vi "WSVCAP SHL FPGA TL Top Level.vi"() -> ()   [LabVIEW 2012]
uses:
  Type Defs/WSVCAP SHL State.ctl
  Type Defs/WSVCAP SHL Transaction Enum.ctl
  Type Defs/WSVCAP SHL Communication Loop State.ctl
  Type Defs/WSVCAP SHL FIFO Operation Enum.ctl
  Type Defs/WSVCAP SHL Operation Step Enum.ctl
  Type Defs/WSVCAP SHL Procedure Step Enum.ctl
  Type Defs/WSVCAP SHL Transaction Step Enum.ctl
  <vilib>/Platform/TimedLoop/XDataNode/timing_clust.ctl
  <vilib>/Platform/TimedLoop/XDataNode/nitl_modes.ctl
  <vilib>/Platform/TimedLoop/XDataNode/wakeup.ctl
  WSVCAP Shell FPGA Low Level/WSVCAP SHL FPGA LL RFFE Debug Global.vi
  WSVCAP Shell FPGA Low Level/WSVCAP SHL FPGA LL SPI Debug Global.vi
  WSVCAP Shell FPGA Low Level/WSVCAP SHL FPGA LL I2C Debug Global.vi
  <vilib>/Platform/TimedLoop/XDataNode/XDataNode.xnode
  <vilib>/Platform/TimedLoop/XDataNode/XDNodeRunTimeDep.lvlib
panel:
  in  "Stop Cycle":bool
  out "Cycle Count":u64
  in  "Socket Mask":u64=1 format="%012x"
  in  "Display CH (1-48)":i32=1 min=1 max=48 step=1
  out "Status":i32
  out "Read Data":u64
  in  "Transaction":T1
  in  "Bytes to Write":u8=8
  in  "Sub Address":u8=1 format="%02x"
  in  "Ack Read Status":bool
  out "Read Status Flag":bool
  in  "Exit":bool
  out "Waveform Chart":cluster{i16, i16, i16, i16}(graph)
  in  "Wait Ticks":u32=20
  in  "Slave Address":u8=1 format="%02x"
  in  "Bytes to Read":u8=8
  in  "Start":bool
  in  "Cmd":T2
  in  "Ack Read":bool
  out "Read Flag":bool
  in  "Write Flag":bool
  in  "Write Data":u64
  # "Control"
  # "I2C Configuration Parameters"
  # "Host Data Transfer"
  # "Command Type"
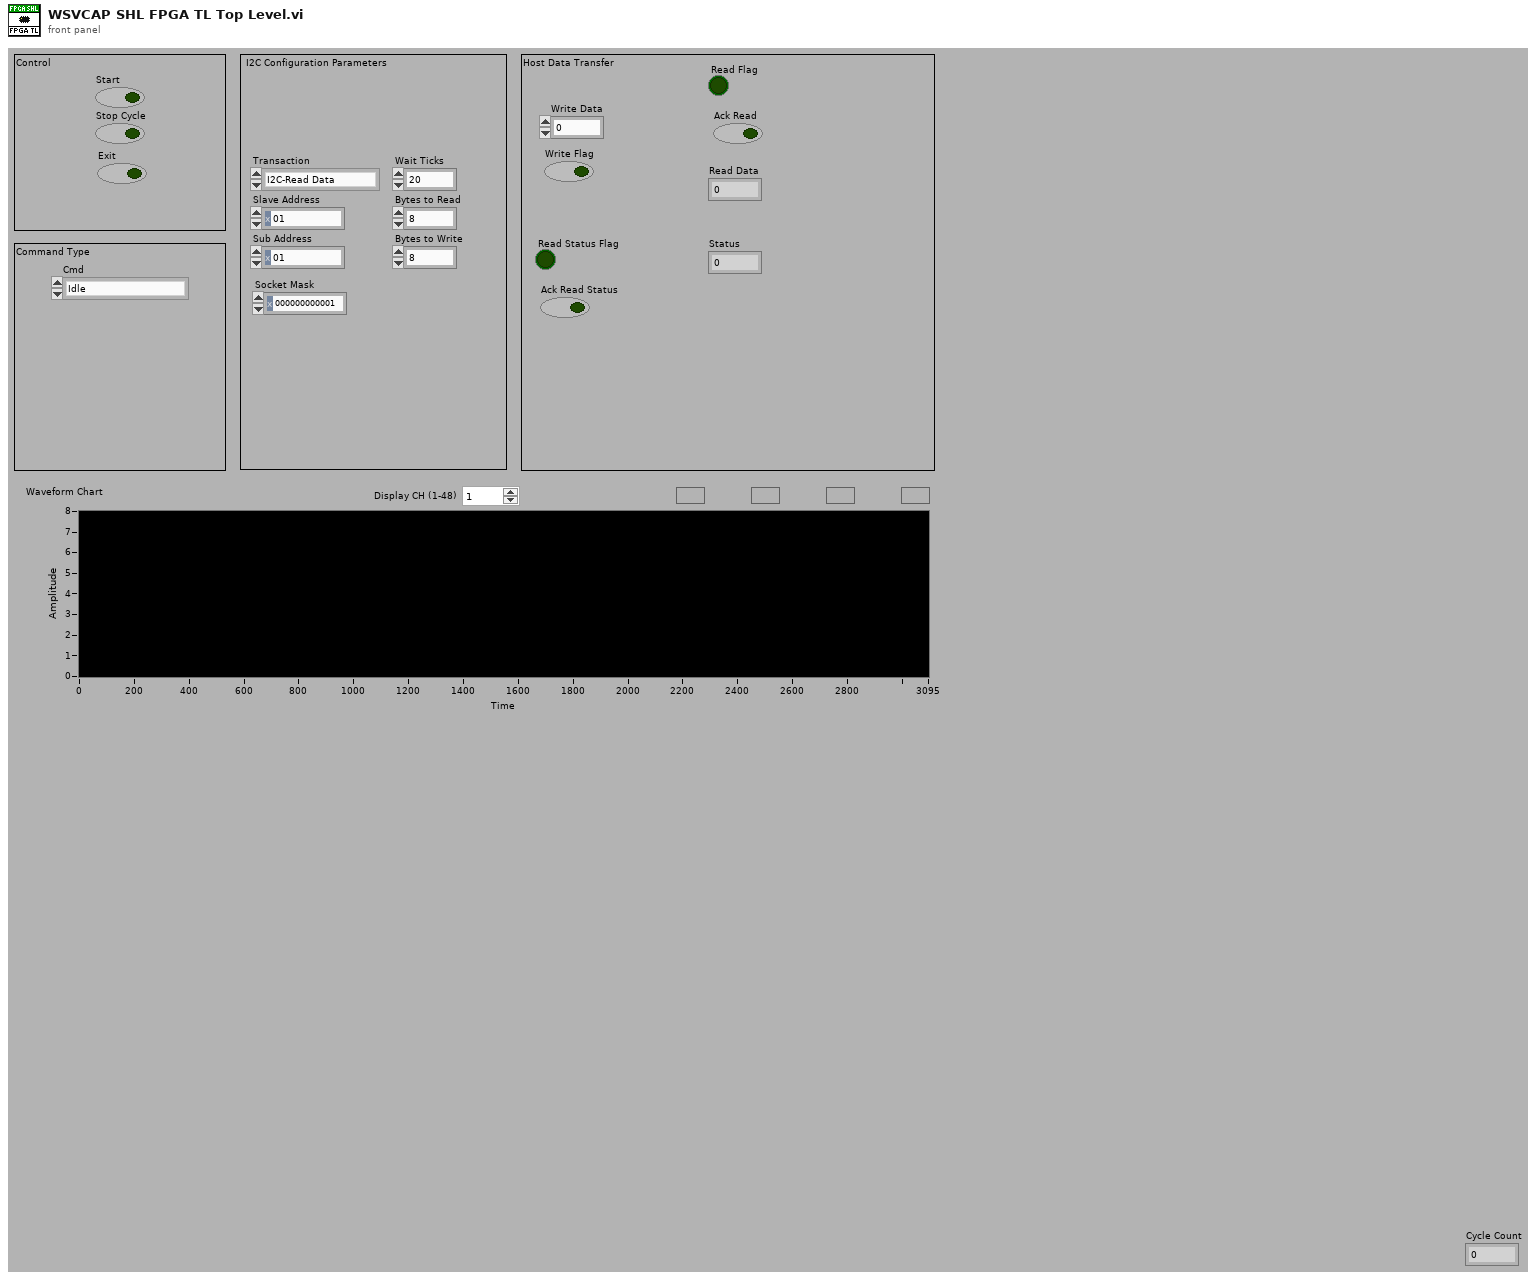
[diagram p1: front panel]
types:
  T1 = typedef "WSVCAP SHL Transaction Enum.ctl" = enum16{"I2C-Read Data", "I2C-Write Data", "SPI-Write/Read Data", "RFFE-Ext Write", "RFFE-Ext Read"}
  T2 = typedef "WSVCAP SHL State.ctl" = enum8{"Idle", "Transfer Data"}
  T3 = typedef "WSVCAP SHL Communication Loop State.ctl" = enum8{"Idle", "Initialize", "Pre-Transmission", "Transmit Data", "Post Transmition", "Operation Complete"}
  T4 = typedef "WSVCAP SHL FIFO Operation Enum.ctl" = enum16{"Create FIFO/Memory", "Get Write FIFO Status", "Get Read FIFO Status", "Put Element in Write", "Put Element in Read", "Get Element from Write", "Get Element from Read"}
  T5 = typedef "WSVCAP SHL Procedure Step Enum.ctl" = enum16{"I2C Start/Stop - 1: Set Clock Low", "I2C Start/Stop - 2: Wait", "I2C Start/Stop - 3: Set Data I", "I2C Start/Stop - 4: Wait", "I2C Start/Stop - 5: Set Clock High", "I2C Start/Stop - 6: Wait", "I2C Start/Stop - 7: Set Data II", "I2C Start/Stop - 8: Wait", "I2C Start/Stop - 9: Set Clock Low", "I2C Start/Stop - 10: Wait", "I2C Read ACK - 1: Set Clock High", "I2C Read ACK - 2: Wait", "I2C Read ACK - 3: Read ACK Bit", "I2C Read ACK - 4: Wait", "I2C Read ACK - 5: Set Clock Low", "I2C Read ACK - 6: Wait", "I2C Write ACK - 1: Write ACK Bit", "I2C Write ACK - 2: Wait", "I2C Write ACK - 3: Set Clock High", "I2C Write ACK - 4: Wait", "I2C Write ACK - 5: Set Clock Low", "I2C Write ACK - 6: Wait", "I2C Write ACK - 7: Set Data Low", "I2C Send Add - 1: Reset Bits Remaining", "I2C Send Add - 2: Set Data Bit", "I2C Send Add - 3: Wait", "I2C Send Add - 4: Set Clock High", "I2C Send Add - 5: Wait", "I2C Send Add - 6: Set Clock Low", "I2C Send Add - 7: Wait", "I2C Send Add - 8: Check Bits Remaining", "I2C Send Data - 1: Reset Bits Remaining", "I2C Send Data - 2: Load Write Bit from FIFO", "I2C Send Data - 3: Set Data Bit", "I2C Send Data - 4: Wait", "I2C Send Data - 5: Set Clock High", "I2C Send Data - 6: Wait", "I2C Send Data - 7: Set Clock Low", "I2C Send Data - 8: Wait", "I2C Send Data - 9: Check Bits Remaining", "I2C Receive Data - 1: Reset Bits Remaining", "I2C Receive Data - 2: Wait", "I2C Receive Data - 3: Set Clock High", "I2C Receive Data - 4: Wait", "I2C Receive Data - 5: Read Data Bit", "I2C Receive Data - 6: Wait", "I2C Receive Data - 7: Set Clock Low", "I2C Receive Data - 8: Wait", "I2C Receive Data - 9: Check Bits Remaining", "SPI Clear Lines - 1:Clear", "SPI Send/Receive - 1: Load SDA - Clock Low", "SPI Send/Receive - 2: Wait", "SPI Send/Receive - 3: Load DATO - Clock High", "SPI Send/Receive - 4: Wait", "SPI Wait CMD Delay - 1:Wait", "RFFE Send SSC - 1:Set Low", "RFFE Send SSC - 2:Wait", "RFFE Send SSC - 3:Set SDA High", "RFFE Send SSC - 4:Wait", "RFFE Send SSC - 5:Set SDA Low", "RFFE Send SSC - 6:Wait", "RFFE Send Data - 1:Set SCL High", "RFFE Send Data - 2:Wait", "RFFE Send Data - 3:Set SCL Low", "RFFE Send Data - 4:Wait", "RFFE Send Data - 5:Set SCL High (P)", "RFFE Send Data - 6:Wait", "RFFE Send Data - 7:Set SCL Low (P)", "RFFE Send Data - 8:Wait", "RFFE Send Data - 9:Set SCL High (BP)", "RFFE Send Data - 10:Wait", "RFFE Send Data - 11:Set SCL Low (BP)", "RFFE Send Data - 12:Wait", "RFFE Receive Data - 1:Set SCL High", "RFFE Receive Data - 2:Wait", "RFFE Receive Data - 3:Set SCL Low", "RFFE Receive Data - 4:Wait", "RFFE Receive Data - 5:Set SCL High (BP)", "RFFE Receive Data - 6:Wait", "RFFE Receive Data - 7:Set SCL Low (BP)", "RFFE Receive Data - 8:Wait", "RFFE Wait CMD Delay - 1:Wait", "RFFE Clear Lines - 1:Clear"}
  T6 = typedef "WSVCAP SHL Operation Step Enum.ctl" = enum16{"I2C Send Slave Add - A: Send Start Sequence", "I2C Send Slave Add - B: Load Address Byte", "I2C Send Slave Add - C: Send Address Byte", "I2C Send Slave Add - D: Read Slave ACK", "I2C Send Sub Add - A: Load Sub Address", "I2C Send Sub Add - B: Send Address Byte", "I2C Send Sub Add - C: Read Slave ACK", "I2C Send Data - A: Get Byte from FIFO", "I2C Send Data - B: Send Data Byte", "I2C Send Data - C: Read Slave ACK", "I2C Send Data - D: Send Stop Sequence", "I2C Read Data - A: Load Bytes to Read", "I2C Read Data - B: Receive Byte", "I2C Read Data - C: Write Master ACK", "I2C Read Data - D: Send Stop Sequence", "SPI Write/Read - A: SPI-Clear Lines", "SPI Write/Read - B: SPI-Send/Receive Data", "SPI Write/Read - C: SPI-Wait CMD Delay", "SPI Write/Read - D:SPI-Clear Lines", "RFFE Read Data - A: Send SSC", "RFFE Read Data - B: Send CMD Frame", "RFFE Read Data - C: Receive Byte", "RFFE Write Data - A: Send SSC", "RFFE Write Data - B: Send Data", "RFFE Write Data - C: Wait CMD Delay", "RFFE Write Data - D: Clear Lines"}
  T7 = typedef "WSVCAP SHL Transaction Step Enum.ctl" = enum16{"I2C Write - I:Send Slave Address", "I2C Write - II:Send Sub Address", "I2C Write - III:Send Data Bytes", "I2C Read - I:Send Slave Address (W)", "I2C Read - II:Send Sub Address", "I2C Read - III:Send Slave Address (R)", "I2C Read - IV:Read Data Bytes", "SPI Write/Read - I:SPI-Write/Read Data", "RFFE Ext Write - I.Write Data", "RFFE Ext Read - I:Read Data"}
  T8 = typedef "XDNodeRunTimeDep.lvlib/timing_clust.ctl" = cluster{"Expected End [f-1]":u64, "Actual End [f-1]":u64, "Finished Late? [f-1]":bool, "Expected End [i-1]":u64, "Actual End [i-1]":u64, "Finished Late? [i-1]":bool, "Expected Start [i]":u64, "Actual Start [i]":u64, "Expected Start [f]":u64, "Actual Start [f]":u64, "Source Name":string, "Structure Name":string, "Period":i64, "Deadline":i64, "Offset":i64, "Start":i64, "Priority":i32, "Timeout":i32, "Mode":T9, "Wakeup Reason":T10, "Error":errorcluster, "Source Type":string, "Secondary Source Type":string, "Global End Time":u64, "Global Start Time":u64, "Frame Duration":u64, "Iteration Duration":u64, "Assigned CPU":i32, "I/O Scan Engine Mode":u32}
  T9 = typedef "XDNodeRunTimeDep.lvlib/nitl_modes.ctl" = enum32{"No Change", "Process missed periods, maintain original phase", "Discard missed periods, maintain original phase", "Process missed periods, ignore original phase", "Discard missed periods, ignore original phase"}
  T10 = typedef "XDNodeRunTimeDep.lvlib/wakeup.ctl" = enum32{"Normal", "Aborted", "Asynchronous wakeup", "Timing source error", "Timed loop error", "Timeout"}
  T11 = typedef "WSVCAP SHL Transaction Cluster.ctl" = cluster{"Transaction":T1, "Write Byte":u8, "Write Bits Remaining":u8, "Read Bits Remaining":u8, "Read Bytes Remaining":u8, "Wait Ticks Remaining":u32, "Slave Address":u8, "Bytes to Read":u8, "Bytes to Write":u8, "Sub Address":u8, "Socket Mask":u64, "Write CMD [1-4]":u8, "Write Bit Index [0-39]":u8, "CMD Delay (Ticks)":u32, "Commands per Cycle [1-4]":u8, "CMD Length [1-48]":u8, "Cycle Count":u64, "Cycle Mode":bool, "CMD 1 Length (Bits)":u8, "CMD 2 Length (Bits)":u8, "CMD 3 Length (Bits)":u8, "CMD 4 Length (Bits)":u8, "CMD 1 Delay (Ticks)":u32, "CMD 2 Delay (Ticks)":u32, "CMD 3 Delay (Ticks)":u32, "CMD 4 Delay (Ticks)":u32, "CMD 1":u64, "CMD 2":u64, "CMD 3":u64, "CMD 4":u64, "Cycle CMD":u64, "Transaction Step":T7, "Operation Step":T6, "Procedure Step":T5, "Start Operation":bool, "Start Procedure":bool, "Procedure":T12, "Wait Ticks":u32}
  T12 = typedef "WSVCAP SHL Procedure Enum.ctl" = enum16{"None", "I2C-Send Start/Stop Sequence", "I2C-Send Address Byte", "I2C-Send Data Byte", "I2C-Read ACK", "I2C-Receive Byte", "I2C-Write ACK", "SPI-Clear Lines", "SPI-Send/Receive", "SPI-Wait CMD Delay", "RFFE-Clear Lines", "RFFE-Send SSC", "RFFE-Send Data", "RFFE-Receive Data", "RFFE-Wait CMD Delay"}
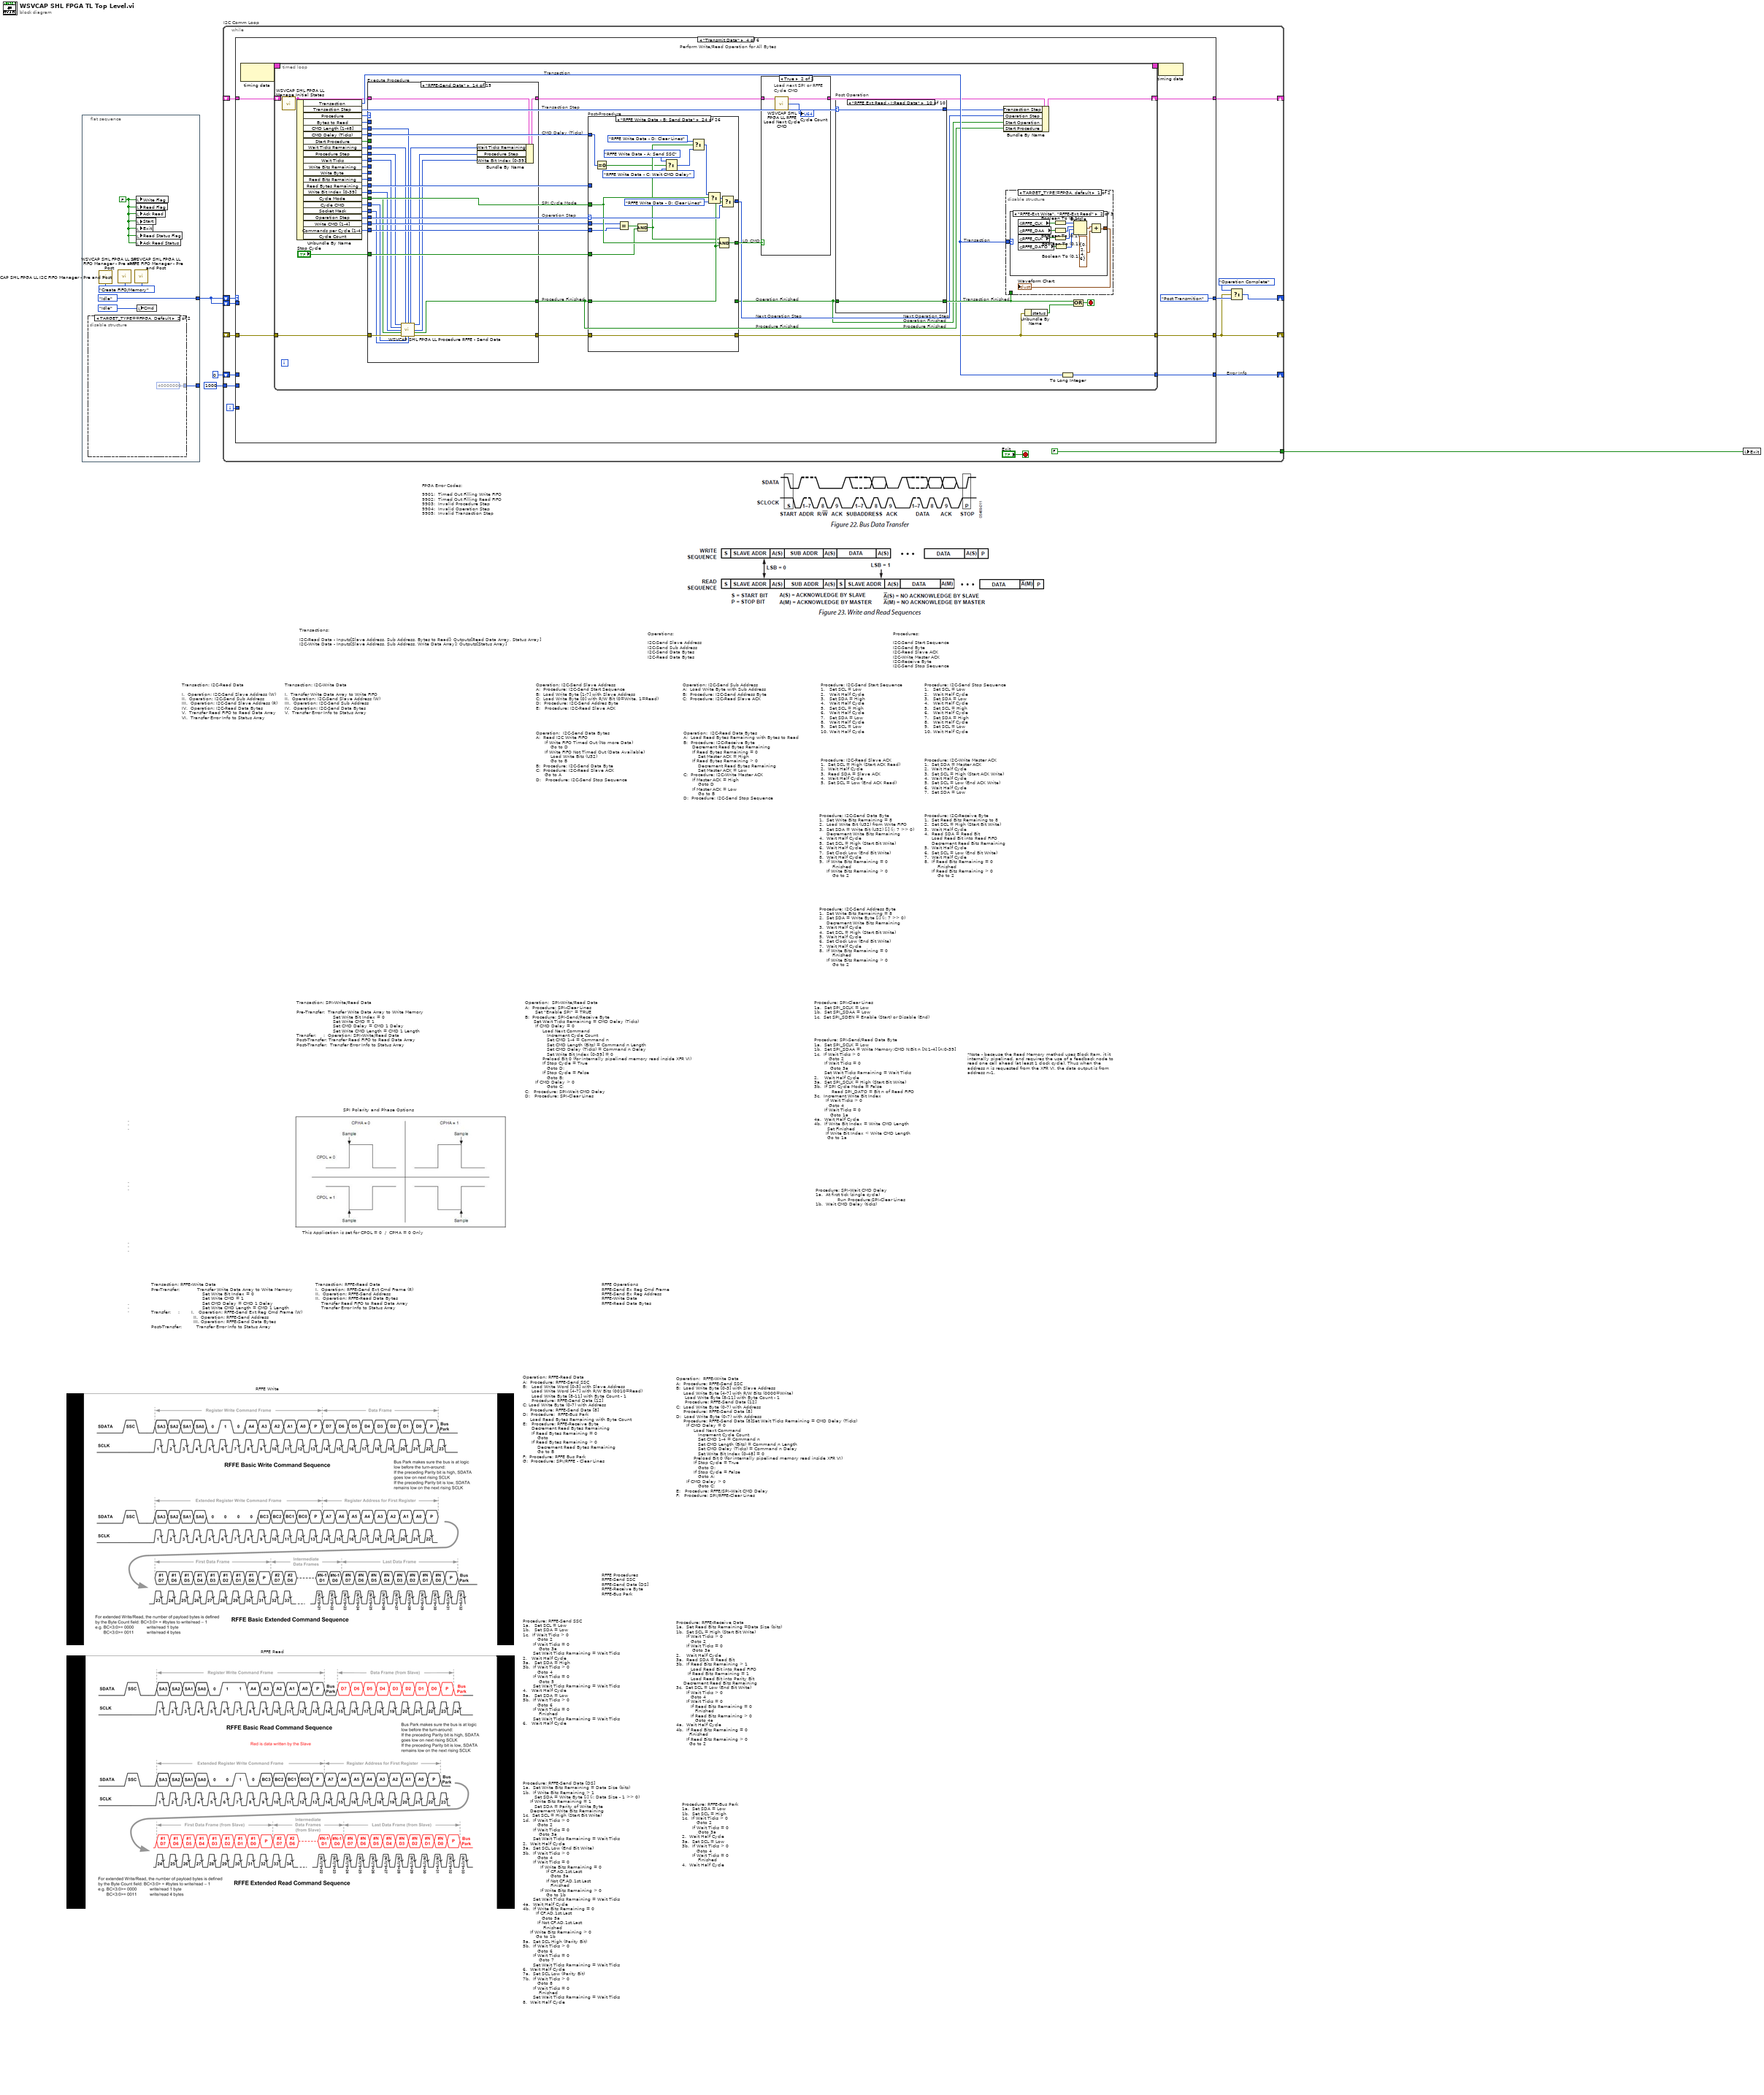
[diagram p0: block diagram]
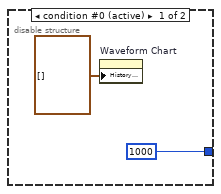
[diagram p2: hidden frame]
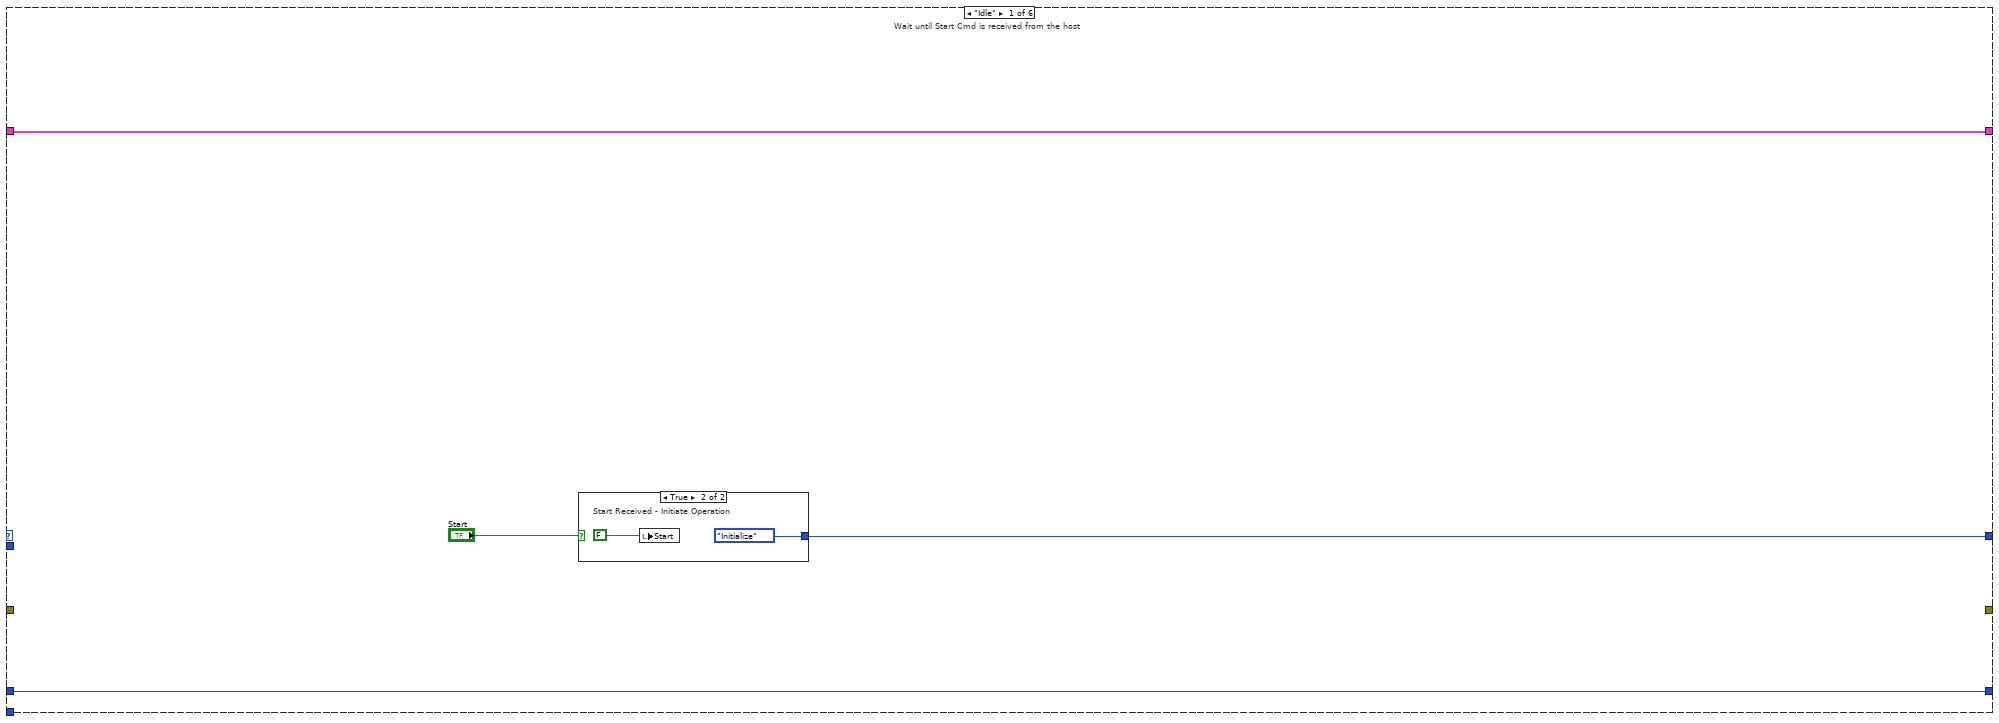
[diagram p3: hidden frame]
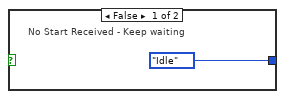
[diagram p4: hidden frame]
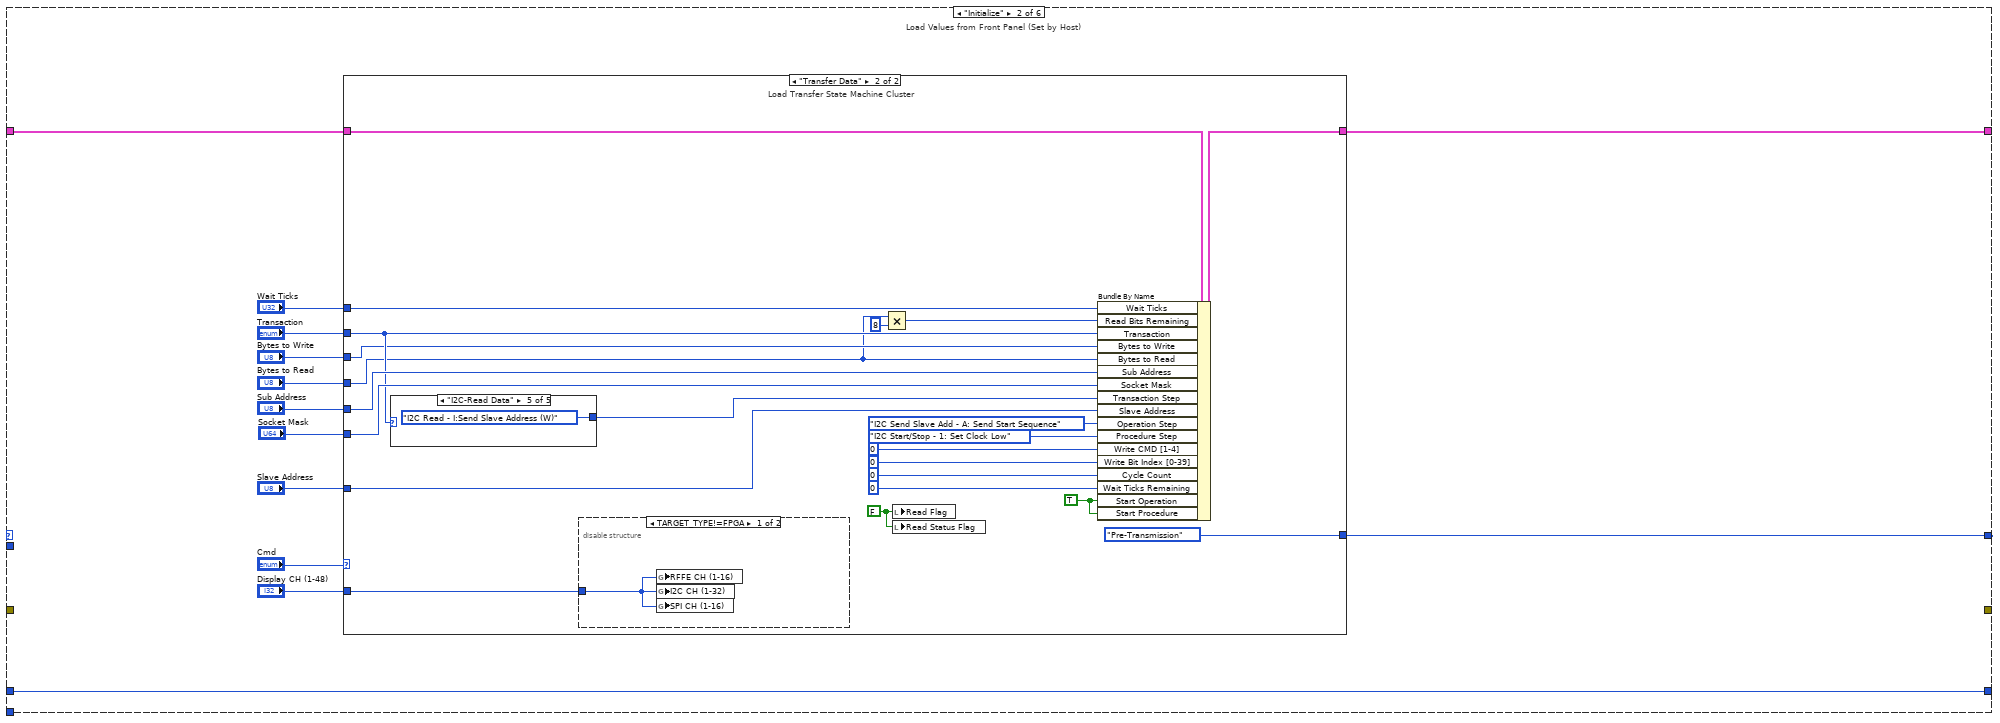
[diagram p5: hidden frame]
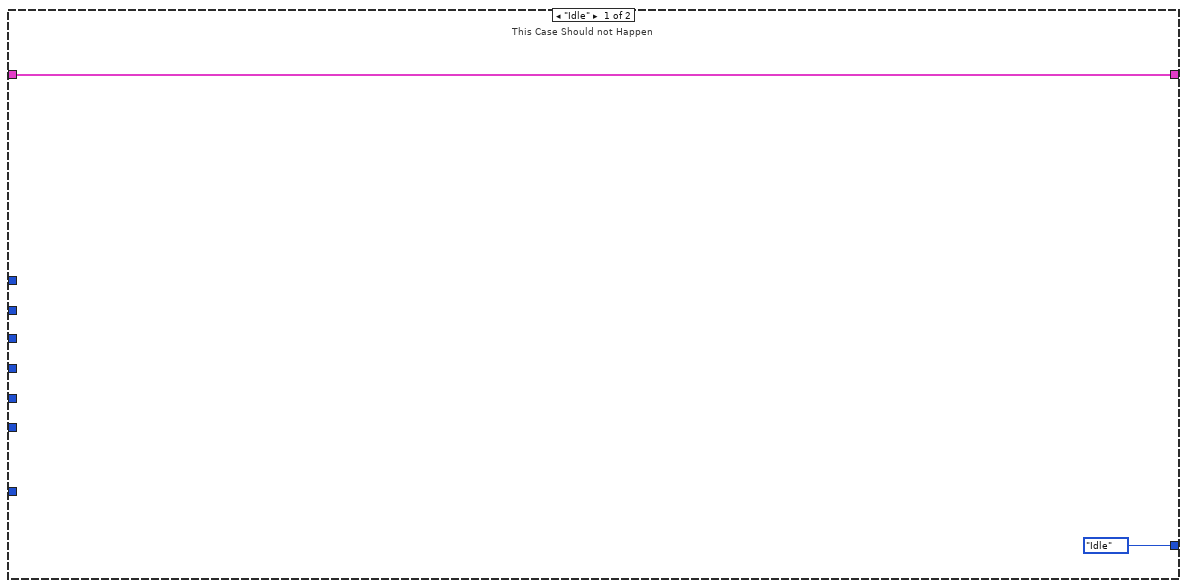
[diagram p6: hidden frame]
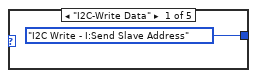
[diagram p7: hidden frame]
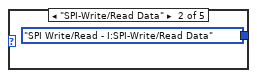
[diagram p8: hidden frame]
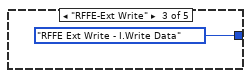
[diagram p9: hidden frame]
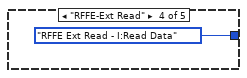
[diagram p10: hidden frame]
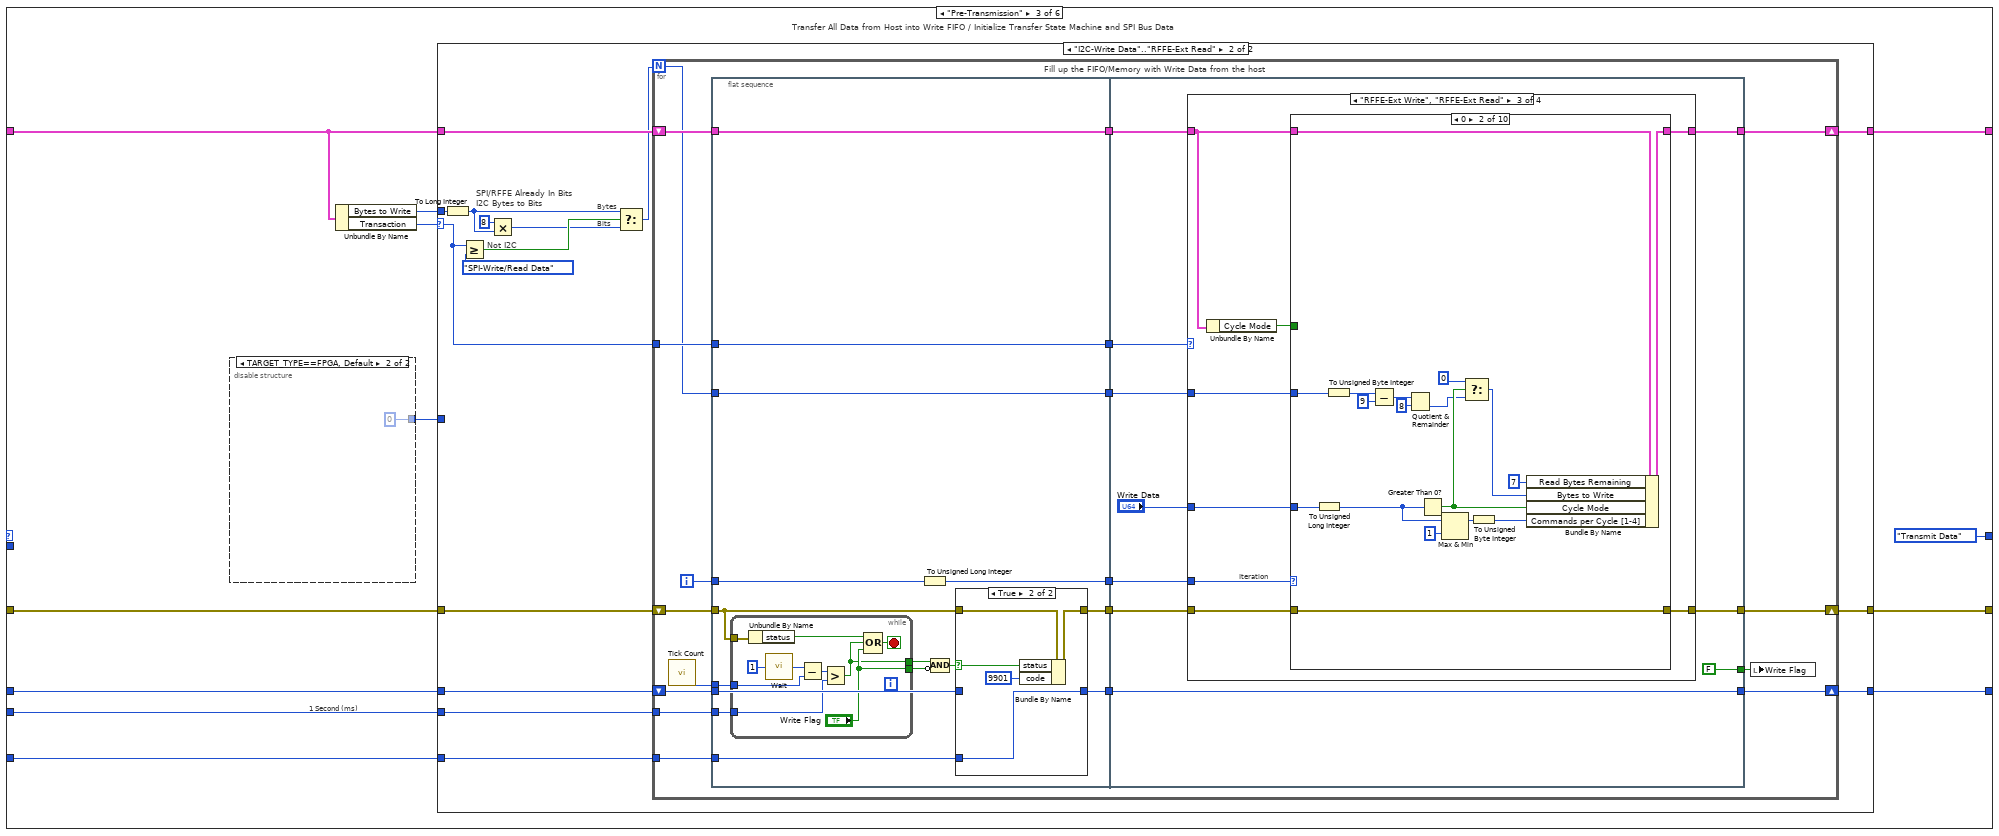
[diagram p12: hidden frame]
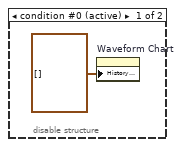
[diagram p13: hidden frame]
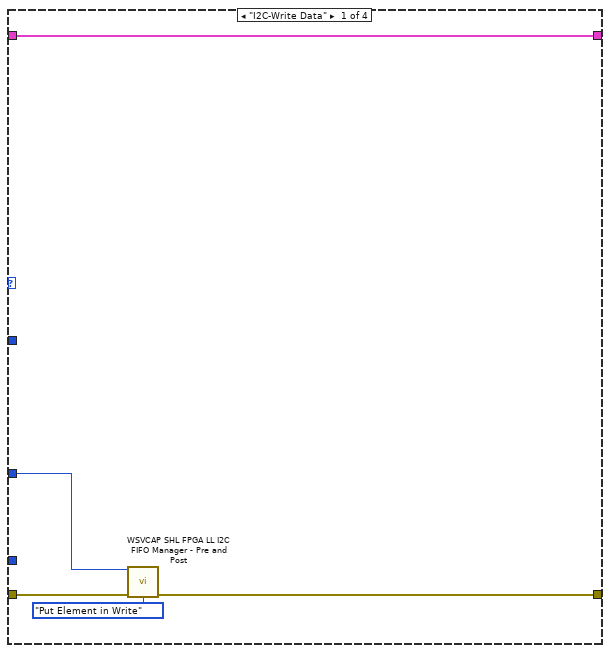
[diagram p16: hidden frame]
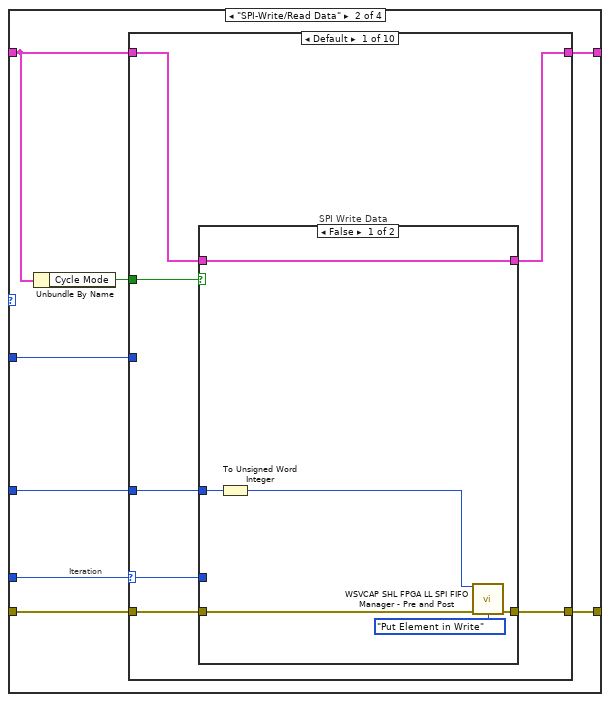
[diagram p17: hidden frame]
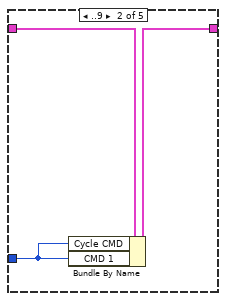
[diagram p19: hidden frame]
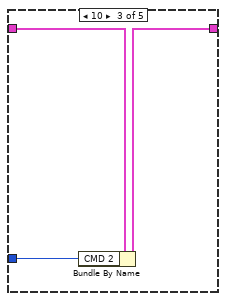
[diagram p20: hidden frame]
diagram:
  # "Operation:  RFFE-Write Data\nA:  Procedure: RFFE-Send SSC\nB:  Load Write Byte [0-3] with Slave Address\n     Load Write Byte [4-7] with R/W Bits (0000=Write)\n      Load Write Byte [8-11] with Byte Count - 1\n      Procedure: RFFE-Send Data [12]\nC:  Load Write Byte (0-7) with Address\n     Procedure: RFFE-Send Data [8]\nD:  Load Write Byte (0-7) with Address\n     Procedure: RFFE-Send Data [8]Set Wait Ticks Remaining = CMD Delay (Ticks)\n       If CMD Delay = 0\n            Load Next Command\n               Increment Cycle Count\n               Set CMD 1-4 = Command n\n               Set CMD Length (Bits) = Command n Length\n               Set CMD Delay (Ticks) = Command n Delay\n               Set Write Bit Index [0-48] = 0\n            Preload Bit 0 (for internally pipelined memory read inside XFR VI)\n            If Stop Cycle = True\n               Goto D:\n            If Stop Cycle = False\n               Goto A:\n       If CMD Delay > 0\n               Goto C:\nE:   Procedure: RFFE/SPI-Wait CMD Delay          \nF:   Procedure: SPI/RFFE-Clear Lines"
  # "Operation: RFFE-Read Data\nA:  Procedure: RFFE-Send SSC\nB:   Load Write Word [0-3] with Slave Address\n      Load Write Word [4-7] with R/W Bits (0010=Read)\n      Load Write Byte [8-11] with Byte Count - 1\n      Procedure: RFFE-Send Data [12]\nC: Load Write Byte (0-7) with Address\n     Procedure: RFFE-Send Data [8]\nD:  Procedure:  RFFE-Bus Park\n     Load Read Bytes Remaining with Byte Count\nE:   Procedure: RFFE-Receive Byte\n      Decrement Read Bytes Remaining\n      If Read Bytes Remaining = 0\n          Goto\n      If Read Bytes Remaining > 0\n          Decrement Read Bytes Remaining\n          Go to B\nF:  Procedure: RFFE Bus Park\nG:  Procedure: SPI/RFFE - Clear Lines"
  # "RFFE Write"
  # "RFFE Read"
  # "Transaction: RFFE-Write Data\nPre-Transfer:            Transfer Write Data Array to Write Memory\n                                   Set Write Bit Index = 0\n                                   Set Write CMD = 1\n                                   Set CMD Delay = CMD 1 Delay\n                                   Set Write CMD Length = CMD 1 Length\nTransfer:     :        I.   Operation: RFFE-Send Ext Reg Cmd Frame (W)\n                             II.  Operation: RFFE-Send Address\n                             III. Operation: RFFE-Send Data Bytes\nPost-Transfer:          Transfer Error Info to Status Array"
  # "Procedure: RFFE-Send Data [DS]\n1a.  Set Write Bits Remaining = Data Size (bits)\n1b.  If Write Bits Remaining > 1\n        Set SDA = Write Byte [i] (i: Data Size - 1 >> 0)\n     If Write Bits Remaining = 1\n        Set SDA = Parity of Write Byte\n     Decrement Write Bits Remaining\n1c.  Set SCL = High (Start Bit Write)\n1d.  If Wait Ticks > 0\n          Goto 2\n       If Wait Ticks = 0 \n           Goto 3a\n       Set Wait Ticks Ramaining = Wait Ticks\n2.  Wait Half Cycle\n3a.  Set SCL Low (End Bit Write)\n3b.  If Wait Ticks > 0\n          Goto 4\n       If Wait Ticks = 0 \n            If Write Bits Remaining = 0\n                If CF,AD,1st,Last\n                   Goto 5a\n                If Not CF,AD,1st,Last\n                   Finished\n            If Write Bits Remaining > 0\n                Go to 1b\n       Set Wait Ticks Ramaining = Wait Ticks\n4a.  Wait Half Cycle\n4b.  If Write Bits Remaining = 0\n         If CF,AD,1st,Last\n             Goto 5a\n          If Not CF,AD,1st,Last\n              Finished\n     If Write Bits Remaining > 0\n         Go to 1b\n5a.  Set SCL High (Parity Bit)\n5b.  If Wait Ticks > 0\n          Goto 6\n       If Wait Ticks = 0 \n           Goto 7\n       Set Wait Ticks Ramaining = Wait Ticks\n6.  Wait Half Cycle\n7a.  Set SCL Low (Parity Bit)\n7b.  If Wait Ticks > 0\n          Goto 8\n       If Wait Ticks = 0 \n           Finished\n       Set Wait Ticks Ramaining = Wait Ticks\n8.  Wait Half Cycle"
  # "Procedure: RFFE-Bus Park\n1a.  Set SDA = Low\n1b.  Set SCL = High\n1c.  If Wait Ticks > 0\n          Goto 2\n       If Wait Ticks = 0 \n           Goto 3a\n2.  Wait Half Cycle\n3a.  Set SCL = Low\n3b.  If Wait Ticks > 0\n          Goto 4\n       If Wait Ticks = 0 \n           Finished\n4.  Wait Half Cycle"
  # "Procedure: RFFE-Send SSC\n1a.   Set SCL = Low\n1b.   Set SDA = Low\n1c.  If Wait Ticks > 0\n          Goto 2\n       If Wait Ticks = 0 \n           Goto 3a\n       Set Wait Ticks Ramaining = Wait Ticks\n2.   Wait Half Cycle\n3a.   Set SDA = High\n3b.  If Wait Ticks > 0\n          Goto 4\n       If Wait Ticks = 0 \n           Goto 5\n       Set Wait Ticks Ramaining = Wait Ticks\n4.   Wait Half Cycle\n5a.   Set SDA = Low\n5b.  If Wait Ticks > 0\n          Goto 6\n       If Wait Ticks = 0 \n           Finished\n       Set Wait Ticks Ramaining = Wait Ticks\n6.   Wait Half Cycle"
  # "Procedure: RFFE-Receive Data\n1a.  Set Read Bits Remaining =Data Size (bits)\n1b.  Set SCL = High (Start Bit Write)\n       If Wait Ticks > 0\n          Goto 2\n       If Wait Ticks = 0 \n           Goto 3a\n2.    Wait Half Cycle\n3a.  Read SDA = Read Bit\n3b.  If Read Bits Remaining > 1\n          Load Read Bit into Read FIFO\n        If Read Bits Remaining = 1\n          Load Read Bit into Parity Bit\n     Decrement Read Bits Remaining\n3c.  Set SCL = Low (End Bit Write)\n       If Wait Ticks > 0\n          Goto 4\n       If Wait Ticks = 0\n          If Read Bits Remaining = 0\n             Finished\n          If Read Bits Remaining > 0\n             Goto 4a\n4a.  Wait Half Cycle\n4b.  If Read Bits Remaining = 0\n         Finished\n       If Read Bits Remaining > 0\n         Go to 2"
  # "RFFE Procedures\nRFFE-Send SSC\nRFFE-Send Data [DS]\nRFFE-Receive Byte\nRFFE-Bus Park"
  # "Transaction: RFFE-Read Data\nI.  Operation: RFFE-Send Ext Cmd Frame (R)\nII.  Operation: RFFE-Send Address\nII.  Operation: RFFE-Read Data Bytes\n    Transfer Read FIFO to Read Data Array\n    Transfer Error Info to Status Array"
  # "RFFE Operations\nRFFE-Send Ex Reg Cmd Frame\nRFFE-Send Ex Reg Address\nRFFE-Write Data\nRFFE-Read Data Bytes"
  # "*Note - because the Read Memory method uses Block Ram, it it internally pipelined, and requires the use of a feedback node to read one call ahead (at least 1 clock cycle). Thus when the address n is requested from the XFR VI, the data output is from address n-1."
  # "SPI Polarity and Phase Options"
  # "Procedure: SPI-Wait CMD Delay\n1a.  At first tick (single cycle)\n               Run Procedure:SPI-Clear Lines\n1b.  Wait CMD Delay (ticks)"
  # "Procedure: SPI-Clear Lines\n1a.  Set SPI_SCLK = Low\n1b.  Set SPI_SDAA = Low\n1c.  Set SPI_SDEN = Enable (Start) or Disable (End)"
  # "This Application is set for CPOL = 0  /  CPHA = 0 Only"
  # "Procedure: SPI-Send/Read Data Byte\n1a.  Set SPI_SCLK = Low\n1b.  Set SPI_SDAA = Write Memory:CMD N:Bit n [N:1-4] [n:0-39] \n1c.  If Wait Ticks > 0\n          Goto 2\n       If Wait Ticks = 0 \n           Goto 3a\n       Set Wait Ticks Ramaining = Wait Ticks\n2.    Wait Half Cycle\n3a.  Set SPI_SCLK = High (Start Bit Write)\n3b.  If SPI Cycle Mode = False\n            Read SPI_DATO = Bit n of Read FIFO            \n3c.  Increment Write Bit Index\n        If Wait Ticks > 0\n          Goto 4\n       If Wait Ticks = 0 \n           Goto 1a \n4a.  Wait Half Cycle\n4b.  If Write Bit Index = Write CMD Length\n         Set Finished\n        If Write Bit Index < Write CMD Length\n         Go to 1a"
  # ".\n.\n."
  # ".\n.\n."
  # ".\n.\n."
  # ".\n.\n."
  # "Operation:  SPI-Write/Read Data\nA:  Procedure: SPI-Clear Lines\n       Set \"Enable SPI\" = TRUE \nB:  Procedure: SPI-Send/Receive Byte\n      Set Wait Ticks Remaining = CMD Delay (Ticks)\n       If CMD Delay = 0\n            Load Next Command\n               Increment Cycle Count\n               Set CMD 1-4 = Command n\n               Set CMD Length (Bits) = Command n Length\n               Set CMD Delay (Ticks) = Command n Delay\n               Set Write Bit Index [0-39] = 0\n            Preload Bit 0 (for internally pipelined memory read inside XFR VI)\n            If Stop Cycle = True\n               Goto D:\n            If Stop Cycle = False\n               Goto B:\n       If CMD Delay > 0\n               Goto C:\nC:   Procedure: SPI-Wait CMD Delay          \nD:   Procedure: SPI-Clear Lines"
  # "FPGA Error Codes:\n\n9901:  Timed Out Filling Write FIFO\n9902:  Timed Out Filling Read FIFO\n9903:  Invalid Procedure Step\n9904:  Invalid Operation Step\n9905:  Invalid Transaction Step"
  # "Transaction: SPI-Write/Read Data\n\nPre-Transfer:  Transfer Write Data Array to Write Memory\n                         Set Write Bit Index = 0\n                         Set Write CMD = 1\n                         Set CMD Delay = CMD 1 Delay\n                         Set Write CMD Length = CMD 1 Length\nTransfer:     :  Operation: SPI-Write/Read Data\nPost-Transfer: Transfer Read FIFO to Read Data Array\nPost-Transfer:  Transfer Error Info to Status Array"
  # "Procedure: I2C-Send Address Byte\n1.  Set Write Bits Remaining = 8\n2.  Set SDA = Write Byte [i] (i: 7 >> 0)\n     Decrement Write Bits Remaining\n3.  Wait Half Cycle\n4.  Set SCL = High (Start Bit Write)\n5.  Wait Half Cycle\n6.  Set Clock Low (End Bit Write)\n7.  Wait Half Cycle\n8.  If Write Bits Remaining = 0\n         Finished\n     If Write Bits Remaining > 0\n         Go to 2"
  # "Procedure: I2C-Write Master ACK\n1.  Set SDA = Master ACK\n2.  Wait Half Cycle\n3.  Set SCL = High (Start ACK Write)\n4.  Wait Half Cycle\n5.  Set SCL = Low (End ACK Write)\n6.  Wait Half Cycle\n7.  Set SDA = Low"
  # "Procedure: I2C-Send Start Sequence\n1.   Set SCL = Low\n2.   Wait Half Cycle\n3.   Set SDA = High\n4.   Wait Half Cycle\n5.   Set SCL = High\n6.   Wait Half Cycle\n7.   Set SDA = Low\n8.   Wait Half Cycle\n9.   Set SCL = Low\n10. Wait Half Cycle"
  # "Procedure: I2C-Send Stop Sequence\n1.   Set SCL = Low\n2.   Wait Half Cycle\n3.   Set SDA = Low\n4.   Wait Half Cycle\n5.   Set SCL = High\n6.   Wait Half Cycle\n7.   Set SDA = High\n8.   Wait Half Cycle\n9.   Set SCL = Low\n10. Wait Half Cycle"
  # "Procedure: I2C-Read Slave ACK\n1.  Set SCL = High (Start ACK Read)\n2.  Wait Half Cycle\n3.  Read SDA = Slave ACK\n4.  Wait Half Cycle\n5.  Set SCL = Low (End ACK Read)"
  # "Procedure: I2C-Receive Byte\n1.  Set Read Bits Remaining to 8\n2.  Set SCL = High (Start Bit Write)\n3.  Wait Half Cycle\n4.  Read SDA = Read Bit\n     Load Read Bit into Read FIFO\n     Decrement Read Bits Remaining\n5.  Wait Half Cycle\n6.  Set SCL = Low (End Bit Write)\n7.  Wait Half Cycle\n8.  If Read Bits Remaining = 0\n         Finished\n     If Read Bits Remaining > 0\n         Go to 2"
  # "Procedure: I2C-Send Data Byte\n1.  Set Write Bits Remaining = 8\n2.  Load Write Bit (U32) from Write FIFO\n3.  Set SDA = Write Bit (U32) [i] (i: 7 >> 0)\n     Decrement Write Bits Remaining\n4.  Wait Half Cycle\n5.  Set SCL = High (Start Bit Write)\n6.  Wait Half Cycle\n7.  Set Clock Low (End Bit Write)\n8.  Wait Half Cycle\n9.  If Write Bits Remaining = 0\n         Finished\n     If Write Bits Remaining > 0\n         Go to 2"
  # "Operation:  I2C-Read Data Bytes\nA:  Load Read Bytes Remaining with Bytes to Read\nB:  Procedure: I2C-Receive Byte\n      Decrement Read Bytes Remaining\n      If Read Bytes Remaining = 0\n          Set Master ACK = High\n      If Read Bytes Remaining > 0\n          Decrement Read Bytes Remaining\n          Set Master ACK = Low\nC:  Procedure: I2C-Write Master ACK\n      If Master ACK = High\n          Goto D\n      If Master ACK = Low\n          Go to B\nD:  Procedure: I2C-Send Stop Sequence"
  # "Operation:  I2C-Send Data Bytes\nA:  Read I2C Write FIFO\n      If Write FIFO Timed Out (No more Data)\n          Go to D\n      If Write FIFO Not Timed Out (Data Available)\n          Load Write Bits (U32)\n          Go to B\nB:  Procedure: I2C-Send Data Byte\nC:  Procedure: I2C-Read Slave ACK\n      Go to A\nD:   Procedure: I2C-Send Stop Sequence"
  # "Operation: I2C-Send Sub Address\nA:  Load Write Byte with Sub Address\nB:  Procedure: I2C-Send Address Byte\nC:  Procedure: I2C-Read Slave ACK"
  # "Procedures:\n\nI2C-Send Start Sequence\nI2C-Send Byte\nI2C-Read Slave ACK\nI2C-Write Master ACK\nI2C-Receive Byte\nI2C-Send Stop Sequence"
  # "Transaction: I2C-Write Data\n\nI.  Transfer Write Data Array to Write FIFO\nII.  Operation: I2C-Send Slave Address (W)\nIII.  Operation: I2C-Send Sub Address\nIV.  Operation: I2C-Send Data Bytes\nV.  Transfer Error Info to Status Array"
  # "Transaction: I2C-Read Data\n\nI.  Operation: I2C-Send Slave Address (W)\nII.  Operation: I2C-Send Sub Address\nIII.  Operation: I2C-Send Slave Address (R)\nIV.  Operation: I2C-Read Data Bytes\nV.  Transfer Read FIFO to Read Data Array\nVI.  Transfer Error Info to Status Array"
  # "Transactions:\n\nI2C-Read Data - Inputs[Slave Address, Sub Address, Bytes to Read]; Outputs[Read Data Array, Status Array]\nI2C-Write Data - Inputs[Slave Address, Sub Address, Write Data Array]; Outputs[Status Array]"
  # "Operations:\n\nI2C-Send Slave Address\nI2C-Send Sub Address\nI2C-Send Data Bytes\nI2C-Read Data Bytes"
  # "Operation: I2C-Send Slave Address\nA:  Procedure: I2C-Send Start Sequence\nB:  Load Write Byte [1-7] with Slave Address\nC:  Load Write Byte [0] with R/W Bit (0=Write, 1=Read)\nD:  Procedure: I2C-Send Addres Byte\nE:   Procedure: I2C-Read Slave ACK"
  n1 = flat-sequence {
    tunnel: [WSVCAP_SHL_Communication_Loop_State."Idle" ("Action")] -> w3
    tunnel: [w6] -> _
    frame #0 {
      w5 = WSVCAP_SHL_FIFO_Operation_Enum."Create FIFO/Memory" ("Operation")
      w7 = FALSE ("Done")
      n2 = disable-structure shown="TARGET_TYPE==FPGA, Default" {
        disable-tunnel: [u32 1000 ("x-y") u32 40000000 ("x-y")] -> w6
        frame condition #0 (active) {
          n3 = property on="Waveform Chart" class="WFChart (strict)"("History Data"=cluster{i16, i16, i16, i16}[] []) -> ()  [unwired: 2 in, 2 out]
        }
        frame condition #1 {
        }
      }
      n4 = call "WSVCAP SHL FPGA LL I2C FIFO Manager - Pre and Post.vi"("Operation"=w5) -> ()  [unwired: 12 in, 3 out]
      n5 = call "WSVCAP SHL FPGA LL SPI FIFO Manager - Pre and Post.vi"("Operation"=w5) -> ()  [unwired: 12 in, 3 out]
      n6 = call "WSVCAP SHL FPGA LL RFFE FIFO Manager - Pre and Post.vi"("Operation"=w5) -> ()  [unwired: 12 in, 3 out]
      n7 = local write "Write Flag"(w7) -> ()
      n8 = local write "Read Flag"(w7) -> ()
      n9 = local write "Ack Read"(w7) -> ()
      n10 = local write "Start"(w7) -> ()
      n11 = local write "Exit"(w7) -> ()
      n12 = local write "Read Status Flag"(w7) -> ()
      n13 = local write "Ack Read Status"(w7) -> ()
      n14 = local write "Cmd"(WSVCAP_SHL_State."Idle" ("SPI_CMD_DBG")) -> ()
    }
  }
  n15 = while "I2C Comm Loop" {
    shift-right: [w20] -> _
    shift-left: w3 -> [w27]
    shift-right: [w25] -> _
    shift-left: _ -> [w26]
    tunnel: [FALSE] -> w4
    shift-right: [w19] -> _
    shift-left: _ -> [w22]
    shift-left: w3 -> [w17]
    shift-right: [w16] -> _
    shift-left: 0 -> [w15]
    tunnel: u32 1000 ("x-y") -> [w14]
    i -> [w13]
    stop <- "Exit" stop-if-true
    # "Error Info"
    n16 = case shown="\"Transmit Data\"" w27 {
      tunnel: [w31 w46 WSVCAP_SHL_Communication_Loop_State."Transmit Data" ("Action") WSVCAP_SHL_Communication_Loop_State."Post Transmition" ("Action") WSVCAP_SHL_Communication_Loop_State."Operation Complete" ("Action") WSVCAP_SHL_Communication_Loop_State."Idle" ("Action")] -> w21
      tunnel: w26 -> [w28 w45 w80 w377 w859 w955]
      tunnel: [w28 w44 w79 w376 w858 w955] -> w25
      tunnel: [_ _ w82 w374 w866 _] -> w19
      tunnel: w22 -> [_ _ w87 w375 w867 w960]
      tunnel: w17 -> [_ _ _ _ _ w959]
      tunnel: [w29 w43 w83 w373 w863 _] -> w16
      tunnel: w15 -> [w29 w43 w84 _ w862 w957]
      tunnel: w14 -> [_ _ w86 _ w864 w956]
      tunnel: w13 -> [_ _ w85 _ _ _]
      frame "Idle" {
        # "Wait until Start Cmd is received from the host"
        n17 = case shown="True" "Start" {
          tunnel: [WSVCAP_SHL_Communication_Loop_State."Idle" ("Action") WSVCAP_SHL_Communication_Loop_State."Initialize" ("Action")] -> w31
          frame False {
            # "No Start Received - Keep waiting"
          }
          frame True {
            # "Start Received - Initiate Operation"
            n18 = local write "Start"(FALSE ("SPI_Start")) -> ()
          }
        }
      }
      frame "Initialize" {
        # "Load Values from Front Panel (Set by Host)"
        n19 = case shown="\"Transfer Data\"" "Cmd" {
          tunnel: [WSVCAP_SHL_Communication_Loop_State."Idle" ("Action") WSVCAP_SHL_Communication_Loop_State."Pre-Transmission" ("Action")] -> w46
          tunnel: w45 -> [w48 w69]
          tunnel: [w48 w70] -> w44
          tunnel: "Wait Ticks" -> [_ w56]
          tunnel: "Slave Address" -> [_ w54]
          tunnel: "Sub Address" -> [_ w68]
          tunnel: "Display CH (1-48)" -> [_ w66]
          tunnel: "Transaction" -> [_ w59]
          tunnel: "Bytes to Write" -> [_ w55]
          tunnel: "Bytes to Read" -> [_ w52]
          tunnel: "Socket Mask" -> [_ w67]
          frame "Idle" {
            # "This Case Should not Happen"
          }
          frame "Transfer Data" {
            w53 = FALSE ("Read Flag")
            w57 = TRUE ("Read Flag")
            # "Load Transfer State Machine Cluster"
            n20 = case shown="\"I2C-Read Data\"" w59 {
              tunnel: [WSVCAP_SHL_Transaction_Step_Enum."I2C Write - I:Send Slave Address" ("Transaction Step") WSVCAP_SHL_Transaction_Step_Enum."SPI Write/Read - I:SPI-Write/Read Data" ("Transaction Step") WSVCAP_SHL_Transaction_Step_Enum."RFFE Ext Write - I.Write Data" ("Transaction Step") WSVCAP_SHL_Transaction_Step_Enum."RFFE Ext Read - I:Read Data" ("Transaction Step") WSVCAP_SHL_Transaction_Step_Enum."I2C Read - I:Send Slave Address (W)" ("Transaction Step")] -> w58
              frame "I2C-Write Data" {
              }
              frame "SPI-Write/Read Data" {
              }
              frame "RFFE-Ext Write" {
              }
              frame "RFFE-Ext Read" {
              }
              frame "I2C-Read Data" {
              }
            }
            n21 = disable-structure shown="TARGET_TYPE!=FPGA" {
              disable-tunnel: w66 -> [w77 _]
              frame condition #0 (active) {
                n22 = global write "WSVCAP SHL FPGA LL RFFE Debug Global.vi" "RFFE CH (1-16)"(w77) -> ()
                n23 = global write "WSVCAP SHL FPGA LL I2C Debug Global.vi" "I2C CH (1-32)"(w77) -> ()
                n24 = global write "WSVCAP SHL FPGA LL SPI Debug Global.vi" "SPI CH (1-16)"(w77) -> ()
              }
              frame condition #1 {
              }
            }
            n25 = Multiply(x=w52, y=u8 8) -> (x*y=w50:u8)
            n26 = local write "Read Flag"(w53) -> ()
            n27 = local write "Read Status Flag"(w53) -> ()
            n28 = Bundle By Name(cluster=w69, "Wait Ticks"=w56, "Read Bits Remaining"=w50, "Transaction"=w59, "Bytes to Write"=w55, "Bytes to Read"=w52, "Sub Address"=w68, "Socket Mask"=w67, "Transaction Step"=w58, "Slave Address"=w54, "Operation Step"=WSVCAP_SHL_Operation_Step_Enum."I2C Send Slave Add - A: Send Start Sequence", "Procedure Step"=WSVCAP_SHL_Procedure_Step_Enum."I2C Start/Stop - 1: Set Clock Low", "Write CMD [1-4]"=u8 0, "Write Bit Index [0-39]"=u8 0, "Cycle Count"=u64 0 ("SPI Cycle Count"), "Wait Ticks Remaining"=u32 0, "Start Operation"=w57, "Start Procedure"=w57) -> (w70:T11)
          }
        }
      }
      frame "Pre-Transmission" {
        # "1 Second (ms)"
        # "Transfer All Data from Host into Write FIFO / Initialize Transfer State Machine and SPI Bus Data"
        n29 = disable-structure shown="TARGET_TYPE==FPGA, Default" {
          disable-tunnel: [_ i16 0] -> w78
          frame condition #0 (active) {
            n30 = property on="Waveform Chart" class="WFChart (strict)"("History Data"=cluster{i16, i16, i16, i16}[] []) -> ()  [unwired: 2 in, 2 out]
          }
          frame condition #1 {
          }
        }
        n31 = Unbundle By Name(w80) -> ("Bytes to Write"=w88:u8, "Transaction"=w81:T1)
        n32 = case shown="\"I2C-Write Data\"..\"RFFE-Ext Read\"" w81 {
          selector: w81 -> [_ w103]
          tunnel: w88 -> [_ w98]
          tunnel: [w94 w110] -> w82
          tunnel: w87 -> [w94 w109]
          tunnel: w86 -> [_ w107]
          tunnel: w85 -> [_ w106]
          tunnel: w84 -> [w93 w105]
          tunnel: [w93 w104] -> w83
          tunnel: w80 -> [w92 w100]
          tunnel: [w92 w99] -> w79
          tunnel: w78 -> [_ _]
          frame "I2C-Read Data" {
          }
          frame "I2C-Write Data".."RFFE-Ext Read" {
            # "Bits"
            # "Bytes"
            # "Not I2C"
            # "SPI/RFFE Already In Bits\nI2C Bytes to Bits"
            n33 = To Long Integer(number=w98) -> (32bit integer=w96:i32)
            n34 = Greater Or Equal?(x=w103, y=WSVCAP_SHL_Transaction_Enum."SPI-Write/Read Data" ("Transaction")) -> (x >= y?=w101:bool)
            n35 = Multiply(x=8, y=w96) -> (x*y=w97:i32)
            n36 = Select(t=w96, s=w101, f=w97) -> (s? t:f=w95:i32)
            n37 = for {
              N: w95 -> [w111]
              shift-right: [w128] -> w110
              shift-left: w109 -> [w126]
              tunnel: w103 -> [w124]
              tunnel: w107 -> [w122]
              tunnel: w106 -> [w121]
              shift-right: [w119] -> w104
              shift-left: w105 -> [w120]
              shift-right: [w113] -> w99
              shift-left: w100 -> [w114]
              i -> [w116]
              # "Fill up the FIFO/Memory with Write Data from the host"
              n38 = call "Tick Count"() -> ("Tick Count(mSec)"=w123:u32)
              n39 = flat-sequence {
                tunnel: [w137] -> w127
                tunnel: w126 -> [w138]
                tunnel: [w144] -> w125
                tunnel: w124 -> [w144]
                tunnel: w123 -> [w143]
                tunnel: w122 -> [w142]
                tunnel: w121 -> [w136]
                tunnel: w120 -> [w135]
                tunnel: [w134] -> w118
                tunnel: [w132] -> w117
                tunnel: w116 -> [w133]
                tunnel: [w131] -> w115
                tunnel: w114 -> [w131]
                tunnel: [w130] -> w112
                tunnel: w111 -> [w130]
                tunnel: [FALSE ("SPI_Write Flag")] -> w129
                tunnel: [w170] -> w128
                tunnel: w127 -> [w169]
                tunnel: w125 -> [w168]
                tunnel: [w167] -> w119
                tunnel: w118 -> [w167]
                tunnel: w117 -> [w166]
                tunnel: w115 -> [w165]
                tunnel: [w164] -> w113
                tunnel: w112 -> [w162]
                frame #0 {
                  n40 = while {
                    tunnel: w143 -> [w159]
                    tunnel: w142 -> [w157]
                    tunnel: w138 -> [w156]
                    tunnel: ["Write Flag"] -> w141
                    tunnel: [w152] -> w140
                    stop <- w154 stop-if-true
                    n41 = Unbundle By Name(w156) -> ("status"=w155:bool)
                    n42 = call "Wait"("Count(mSec)"=u32 1 ("Count(Ticks)")) -> ("Tick Count(mSec)"=w160:u32)
                    n43 = Subtract(x=w160, y=w159) -> (x-y=w158:u32)
                    n44 = Greater?(x=w158, y=w157) -> (0:w152:bool)
                    n45 = Compound Arithmetic op=OR(w155, w152, "Write Flag") -> (w154:bool)
                  }
                  n46 = To Unsigned Long Integer(number=w133) -> (unsigned 32bit integer=w132:u32)
                  n47 = Compound Arithmetic op=AND(w140, invert w141) -> (w139:bool)
                  n48 = case shown="True" w139 {
                    selector: w139 -> [_ w150]
                    tunnel: [w146 w149] -> w137
                    tunnel: w138 -> [w146 w151]
                    tunnel: w136 -> [_ w147]
                    tunnel: [w145 w147] -> w134
                    tunnel: w135 -> [w145 _]
                    frame False {
                    }
                    frame True {
                      n49 = Bundle By Name(cluster=w151, "status"=w150, "code"=9901) -> (w149:errorcluster)
                    }
                  }
                }
                frame #1 {
                  n50 = case shown="\"RFFE-Ext Write\", \"RFFE-Ext Read\"" w168 {
                    tunnel: "Write Data" -> [w172 w181 w278 _]
                    tunnel: [w175 w182 w279 w372] -> w170
                    tunnel: w169 -> [w174 w183 w280 w372]
                    tunnel: w166 -> [_ w184 w281 _]
                    tunnel: w165 -> [w173 w179 w276 w371]
                    tunnel: [w173 w180 w277 w371] -> w164
                    tunnel: w162 -> [_ w177 w274 _]
                    frame "I2C-Write Data" {
                      n51 = call "WSVCAP SHL FPGA LL I2C FIFO Manager - Pre and Post.vi"("64 Bit Data In"=w172, "error in (no error)"=w174, "Operation"=WSVCAP_SHL_FIFO_Operation_Enum."Put Element in Write") -> ("error out"=w175:errorcluster)  [unwired: 10 in, 2 out]
                    }
                    frame "SPI-Write/Read Data" {
                      # "Iteration"
                      n52 = Unbundle By Name(w179) -> ("Cycle Mode"=w178:bool)
                      n53 = case shown="Default" w184 {
                        selector: w184 -> [w186 _ _ _ _ _ _ _ _ _]
                        tunnel: w183 -> [w191 w228 w236 w241 w246 w251 w256 w261 w266 w271]
                        tunnel: [w190 w228 w236 w241 w246 w251 w256 w261 w266 w271] -> w182
                        tunnel: w181 -> [w189 w230 w235 w240 w245 w250 w255 w260 w265 w270]
                        tunnel: w179 -> [w188 w227 w238 w243 w248 w253 w258 w263 w268 w273]
                        tunnel: [w187 w229 w237 w242 w247 w252 w257 w262 w267 w272] -> w180
                        tunnel: w178 -> [w185 _ _ _ _ _ _ _ _ _]
                        tunnel: w177 -> [_ w222 _ _ _ _ _ _ _ _]
                        frame Default {
                          # "SPI Write Data"
                          n54 = case shown="False" w185 {
                            tunnel: w191 -> [w197 w199]
                            tunnel: [w196 w199] -> w190
                            tunnel: w189 -> [w192 w198]
                            tunnel: w188 -> [w193 w202]
                            tunnel: [w193 w201] -> w187
                            tunnel: w186 -> [_ w200]
                            frame False {
                              n55 = To Unsigned Word Integer(number=w192) -> (unsigned 16bit integer=w194:u16)
                              n56 = call "WSVCAP SHL FPGA LL SPI FIFO Manager - Pre and Post.vi"("Word In"=w194, "error in (no error)"=w197, "Operation"=WSVCAP_SHL_FIFO_Operation_Enum."Put Element in Write") -> ("error out"=w196:errorcluster)  [unwired: 10 in, 2 out]
                            }
                            frame True {
                              n57 = case shown="Default" w200 {
                                tunnel: [w203 w205 w208 w211 w214] -> w201
                                tunnel: w202 -> [w203 w206 w209 w212 w215]
                                tunnel: w198 -> [_ w204 w207 w210 w213]
                                frame Default {
                                }
                                frame ..9 {
                                n58 = Bundle By Name(cluster=w206, "Cycle CMD"=w204, "CMD 1"=w204) -> (w205:T11)
                                }
                                frame 10 {
                                n59 = Bundle By Name(cluster=w209, "CMD 2"=w207) -> (w208:T11)
                                }
                                frame 11 {
                                n60 = Bundle By Name(cluster=w212, "CMD 3"=w210) -> (w211:T11)
                                }
                                frame 12 {
                                n61 = Bundle By Name(cluster=w215, "CMD 4"=w213) -> (w214:T11)
                                }
                              }
                            }
                          }
                        }
                        frame 0 {
                          w223 = u8 0 ("t")
                          n62 = Unbundle By Name(w227) -> ("Bytes to Read"=w226:u8)
                          n63 = To Unsigned Long Integer(number=w230) -> (unsigned 32bit integer=w225:u32)
                          n64 = To Unsigned Byte Integer(number=w222) -> (unsigned 8bit integer=w220:u8)
                          n65 = Subtract(x=w220, y=u8 9) -> (x-y=w218:u8)
                          n66 = Quotient & Remainder(x=w218, y=u8 8) -> (floor(x/y)=w216:u8)  [unwired: 1 out]
                          n67 = Greater Than 0?(x=w225) -> (x > 0?=w224:bool)
                          n68 = Max & Min(x=w225, y=u32 1) -> (max(x,y)=w231:u32)  [unwired: 1 out]
                          n69 = Select(t=w223, s=w224, f=w226) -> ()  [unwired: 1 out]
                          n70 = Select(t=w223, s=w224, f=w216) -> (s? t:f=w219:u8)
                          n71 = To Unsigned Byte Integer(number=w231) -> (unsigned 8bit integer=w233:u8)
                          n72 = Bundle By Name(cluster=w227, "Bytes to Write"=w219, "Bytes to Read"=w219, "Cycle Mode"=w224, "Commands per Cycle [1-4]"=w233) -> (w229:T11)
                        }
                        frame 1 {
                          n73 = To Unsigned Byte Integer(number=w235) -> (unsigned 8bit integer=w234:u8)
                          n74 = Bundle By Name(cluster=w238, "CMD Length [1-48]"=w234, "CMD 1 Length (Bits)"=w234) -> (w237:T11)
                        }
                        frame 2 {
                          n75 = To Unsigned Byte Integer(number=w240) -> (unsigned 8bit integer=w239:u8)
                          n76 = Bundle By Name(cluster=w243, "CMD 2 Length (Bits)"=w239) -> (w242:T11)
                        }
                        frame 3 {
                          n77 = To Unsigned Byte Integer(number=w245) -> (unsigned 8bit integer=w244:u8)
                          n78 = Bundle By Name(cluster=w248, "CMD 3 Length (Bits)"=w244) -> (w247:T11)
                        }
                        frame 4 {
                          n79 = To Unsigned Byte Integer(number=w250) -> (unsigned 8bit integer=w249:u8)
                          n80 = Bundle By Name(cluster=w253, "CMD 4 Length (Bits)"=w249) -> (w252:T11)
                        }
                        frame 5 {
                          n81 = To Unsigned Long Integer(number=w255) -> (unsigned 32bit integer=w254:u32)
                          n82 = Bundle By Name(cluster=w258, "CMD Delay (Ticks)"=w254, "CMD 1 Delay (Ticks)"=w254) -> (w257:T11)
                        }
                        frame 6 {
                          n83 = To Unsigned Long Integer(number=w260) -> (unsigned 32bit integer=w259:u32)
                          n84 = Bundle By Name(cluster=w263, "CMD 2 Delay (Ticks)"=w259) -> (w262:T11)
                        }
                        frame 7 {
                          n85 = To Unsigned Long Integer(number=w265) -> (unsigned 32bit integer=w264:u32)
                          n86 = Bundle By Name(cluster=w268, "CMD 3 Delay (Ticks)"=w264) -> (w267:T11)
                        }
                        frame 8 {
                          n87 = To Unsigned Long Integer(number=w270) -> (unsigned 32bit integer=w269:u32)
                          n88 = Bundle By Name(cluster=w273, "CMD 4 Delay (Ticks)"=w269) -> (w272:T11)
                        }
                      }
                    }
                    frame "RFFE-Ext Write", "RFFE-Ext Read" {
                      # "Iteration"
                      n89 = Unbundle By Name(w276) -> ("Cycle Mode"=w275:bool)
                      n90 = case shown="0" w281 {
                        selector: w281 -> [w283 _ _ _ _ _ _ _ _ _]
                        tunnel: w280 -> [w288 w325 w333 w338 w343 w348 w353 w358 w363 w368]
                        tunnel: [w287 w325 w333 w338 w343 w348 w353 w358 w363 w368] -> w279
                        tunnel: w278 -> [w286 w327 w332 w337 w342 w347 w352 w357 w362 w367]
                        tunnel: w276 -> [w285 w324 w335 w340 w345 w350 w355 w360 w365 w370]
                        tunnel: [w284 w326 w334 w339 w344 w349 w354 w359 w364 w369] -> w277
                        tunnel: w275 -> [w282 _ _ _ _ _ _ _ _ _]
                        tunnel: w274 -> [_ w320 _ _ _ _ _ _ _ _]
                        frame Default {
                          # "RFFE Write Data"
                          n91 = case shown="False" w282 {
                            tunnel: w288 -> [w294 w296]
                            tunnel: [w293 w296] -> w287
                            tunnel: w286 -> [w289 w295]
                            tunnel: w285 -> [w290 w299]
                            tunnel: [w290 w298] -> w284
                            tunnel: w283 -> [_ w297]
                            frame False {
                              n92 = To Unsigned Word Integer(number=w289) -> (unsigned 16bit integer=w291:u16)
                              n93 = call "WSVCAP SHL FPGA LL RFFE FIFO Manager - Pre and Post.vi"("Word In"=w291, "error in (no error)"=w294, "Operation"=WSVCAP_SHL_FIFO_Operation_Enum."Put Element in Write") -> ("error out"=w293:errorcluster)  [unwired: 10 in, 2 out]
                            }
                            frame True {
                              n94 = case shown="..9" w297 {
                                tunnel: [w300 w302 w305 w308 w311] -> w298
                                tunnel: w299 -> [w300 w303 w306 w309 w312]
                                tunnel: w295 -> [_ w301 w304 w307 w310]
                                frame Default {
                                }
                                frame ..9 {
                                n95 = Bundle By Name(cluster=w303, "Cycle CMD"=w301, "CMD 1"=w301) -> (w302:T11)
                                }
                                frame 10 {
                                n96 = Bundle By Name(cluster=w306, "CMD 2"=w304) -> (w305:T11)
                                }
                                frame 11 {
                                n97 = Bundle By Name(cluster=w309, "CMD 3"=w307) -> (w308:T11)
                                }
                                frame 12 {
                                n98 = Bundle By Name(cluster=w312, "CMD 4"=w310) -> (w311:T11)
                                }
                              }
                            }
                          }
                        }
                        frame 0 {
                          n99 = To Unsigned Long Integer(number=w327) -> (unsigned 32bit integer=w323:u32)
                          n100 = To Unsigned Byte Integer(number=w320) -> (unsigned 8bit integer=w318:u8)
                          n101 = Subtract(x=w318, y=u8 9) -> (x-y=w316:u8)
                          n102 = Quotient & Remainder(x=w316, y=u8 8) -> (floor(x/y)=w314:u8)  [unwired: 1 out]
                          n103 = Greater Than 0?(x=w323) -> (x > 0?=w322:bool)
                          n104 = Max & Min(x=w323, y=u32 1) -> (max(x,y)=w328:u32)  [unwired: 1 out]
                          n105 = Select(t=u8 0, s=w322, f=w314) -> (s? t:f=w317:u8)
                          n106 = To Unsigned Byte Integer(number=w328) -> (unsigned 8bit integer=w330:u8)
                          n107 = Bundle By Name(cluster=w324, "Read Bytes Remaining"=u8 7, "Bytes to Write"=w317, "Cycle Mode"=w322, "Commands per Cycle [1-4]"=w330) -> (w326:T11)
                        }
                        frame 1 {
                          n108 = To Unsigned Byte Integer(number=w332) -> (unsigned 8bit integer=w331:u8)
                          n109 = Bundle By Name(cluster=w335, "CMD Length [1-48]"=w331, "CMD 1 Length (Bits)"=w331) -> (w334:T11)
                        }
                        frame 2 {
                          n110 = To Unsigned Byte Integer(number=w337) -> (unsigned 8bit integer=w336:u8)
                          n111 = Bundle By Name(cluster=w340, "CMD 2 Length (Bits)"=w336) -> (w339:T11)
                        }
                        frame 3 {
                          n112 = To Unsigned Byte Integer(number=w342) -> (unsigned 8bit integer=w341:u8)
                          n113 = Bundle By Name(cluster=w345, "CMD 3 Length (Bits)"=w341) -> (w344:T11)
                        }
                        frame 4 {
                          n114 = To Unsigned Byte Integer(number=w347) -> (unsigned 8bit integer=w346:u8)
                          n115 = Bundle By Name(cluster=w350, "CMD 4 Length (Bits)"=w346) -> (w349:T11)
                        }
                        frame 5 {
                          n116 = To Unsigned Long Integer(number=w352) -> (unsigned 32bit integer=w351:u32)
                          n117 = Bundle By Name(cluster=w355, "CMD Delay (Ticks)"=w351, "CMD 1 Delay (Ticks)"=w351) -> (w354:T11)
                        }
                        frame 6 {
                          n118 = To Unsigned Long Integer(number=w357) -> (unsigned 32bit integer=w356:u32)
                          n119 = Bundle By Name(cluster=w360, "CMD 2 Delay (Ticks)"=w356) -> (w359:T11)
                        }
                        frame 7 {
                          n120 = To Unsigned Long Integer(number=w362) -> (unsigned 32bit integer=w361:u32)
                          n121 = Bundle By Name(cluster=w365, "CMD 3 Delay (Ticks)"=w361) -> (w364:T11)
                        }
                        frame 8 {
                          n122 = To Unsigned Long Integer(number=w367) -> (unsigned 32bit integer=w366:u32)
                          n123 = Bundle By Name(cluster=w370, "CMD 4 Delay (Ticks)"=w366) -> (w369:T11)
                        }
                      }
                    }
                    frame "I2C-Read Data" {
                      # "Can't Happen"
                    }
                  }
                }
              }
              n124 = local write "Write Flag"(w129) -> ()
            }
          }
        }
      }
      frame "Transmit Data" {
        # "Perform Write/Read Operation for All Bytes"
        n125 = node-c288() -> (w379:T8)  [unwired: 1 out]
        n126 = timed-loop {
          timing-out: [_] -> w378
          timing: w379 -> [_]
          shift-right: [w405] -> w376
          shift-left: w377 -> [w413]
          tunnel: w375 -> [w410]
          tunnel: [w407] -> w374
          tunnel: [w417] -> w373
          stop <- w418 stop-if-true
          # "LD CMD"
          # "Transaction"
          # "Transaction"
          # "Transaction Finished"
          # "Procedure Finished"
          # "Next Operation Step"
          # "Operation Finished"
          # "Procedure Finished"
          # "Operation Finished"
          # "Next Operation Step"
          # "Procedure Finished"
          # "Operation Step"
          # "SPI Cycle Mode"
          # "CMD Delay (Ticks)"
          # "Transaction Step"
          n127 = call "WSVCAP SHL FPGA LL Manage Initial States.vi"("Transfer Cluster In"=w413) -> ("Transfer Cluster Out"=w411:T11)  [unwired: 14 in]
          n128 = Unbundle By Name(w411) -> ("Transaction"=w415:T1, "Transaction Step"=w414:T7, "Procedure"=w412:T12, "Bytes to Read"=w382:u8, "CMD Length [1-48]"=w390:u8, "CMD Delay (Ticks)"=w389:u32, "Start Procedure"=w400:bool, "Wait Ticks Remaining"=w399:u32, "Procedure Step"=w398:T5, "Wait Ticks"=w397:u32, "Write Bits Remaining"=w396:u8, "Write Byte"=w395:u8, "Read Bits Remaining"=w393:u8, "Read Bytes Remaining"=w381:u8, "Write Bit Index [0-39]"=w391:u8, "Cycle Mode"=w388:bool, "Cycle CMD"=w392:u64, "Socket Mask"=w394:u64, "Operation Step"=w383:T6, "Write CMD [1-4]"=w384:u8, "Commands per Cycle [1-4]"=w385:u8)  [unwired: 1 out]
          n129 = case "Execute Procedure" shown="\"RFFE-Send Data\"" w412 {
            tunnel: w410 -> [w618 w633 w647 w660 w671 w686 w699 w707 w723 w742 w765 w772 w785 w801 w818]
            tunnel: [w618 w632 w646 w659 w670 w685 w698 w706 w722 w741 w764 w771 w784 w800 w817] -> w409
            tunnel: [TRUE ("Finished") w631 w640 w658 w669 w680 w697 TRUE ("Finished") w710 w730 w755 TRUE ("Finished") w776 w786 w808] -> w402
            tunnel: w411 -> [w619 w628 w645 w657 w667 w684 w691 w701 w721 w734 w758 w773 w783 w799 w816]
            tunnel: [w619 w629 w644 w656 w668 w683 w690 w701 w720 w733 w757 w773 w782 w798 w815] -> w387
            tunnel: w389 -> [_ _ _ _ _ _ _ _ _ w736 w760 _ _ _ _]
            tunnel: w400 -> [_ _ _ _ _ _ _ _ _ w739 w748 _ _ _ w804]
            tunnel: w399 -> [_ w624 w642 w652 w662 w682 w694 _ w714 w738 w762 _ w779 w793 w811]
            tunnel: w398 -> [_ w626 w638 w651 w665 w676 w693 _ w715 _ _ _ w780 w794 w812]
            tunnel: w397 -> [_ w622 w637 w650 w664 w675 w692 _ w708 _ _ _ w775 w788 w806]
            tunnel: w394 -> [_ w621 w634 w648 w663 w672 w695 w702 w719 w735 w759 w770 w781 w797 w814]
            tunnel: w396 -> [_ _ w636 w649 _ _ _ _ _ _ _ _ _ _ _]
            tunnel: w395 -> [_ _ w635 _ _ _ _ _ _ _ _ _ _ _ _]
            tunnel: w393 -> [_ _ _ _ _ w674 _ _ _ _ _ _ _ _ w805]
            tunnel: w381 -> [_ _ _ _ _ w673 w687 _ _ _ _ _ _ _ w803]
            tunnel: w392 -> [_ _ _ _ _ _ _ _ w718 _ _ _ _ w796 w813]
            tunnel: w388 -> [_ _ _ _ _ _ _ _ w717 _ _ _ _ w795 _]
            tunnel: w391 -> [_ _ _ _ _ _ _ _ w716 _ _ _ _ w787 _]
            tunnel: w390 -> [_ _ _ _ _ _ _ _ w713 _ _ _ _ w792 _]
            tunnel: "Stop Cycle" -> [_ _ _ _ _ _ _ _ _ w726 w751 _ _ _ _]
            tunnel: w385 -> [_ _ _ _ _ _ _ _ _ w728 w753 _ _ _ _]
            tunnel: w384 -> [_ _ _ _ _ _ _ _ _ w725 w750 _ _ _ _]
            tunnel: w383 -> [_ w620 _ _ _ _ _ w700 _ _ _ _ _ _ _]
            tunnel: w382 -> [_ _ _ _ _ _ _ _ _ _ _ _ _ _ _]
            frame "None" {
            }
            frame "I2C-Send Start/Stop Sequence" {
              n130 = Equal?(x=w620, y=WSVCAP_SHL_Operation_Step_Enum."I2C Send Slave Add - A: Send Start Sequence" ("Operation Step")) -> (x = y?=w627:bool)
              n131 = call "WSVCAP SHL FPGA LL Procedure I2C - Send Start or Stop Sequence.vi"("Procedure Step"=w626, "Wait Ticks Remaining"=w624, "I2C Wait Ticks"=w622, "error in (no error)"=w633, "Type (T:Start; F:Stop)"=w627, "Socket Mask"=w621) -> ("Wait Ticks Remaining Out"=w623:u32, "Procedure Step Out"=w625:T5, "Finished"=w631:bool, "error out"=w632:errorcluster)  [unwired: 6 in]
              n132 = Bundle By Name(cluster=w628, "Wait Ticks Remaining"=w623, "Procedure Step"=w625) -> (w629:T11)
            }
            frame "I2C-Send Address Byte" {
              n133 = call "WSVCAP SHL FPGA LL Procedure I2C - Send Address Byte.vi"("Procedure Step"=w638, "Wait Ticks Remaining"=w642, "I2C Wait Ticks"=w637, "Write Bits Remaining"=w636, "Write Byte"=w635, "error in (no error)"=w647, "Socket Mask"=w634) -> ("Wait Ticks Remaining Out"=w641:u32, "Procedure Step Out"=w643:T5, "Write Bits Remaining Out"=w639:u8, "Finished"=w640:bool, "error out"=w646:errorcluster)  [unwired: 4 in]
              n134 = Bundle By Name(cluster=w645, "Wait Ticks Remaining"=w641, "Procedure Step"=w643, "Write Bits Remaining"=w639) -> (w644:T11)
            }
            frame "I2C-Send Data Byte" {
              n135 = call "WSVCAP SHL FPGA LL I2C Procedure - Send Data Byte.vi"("Procedure Step"=w651, "Wait Ticks Remaining"=w652, "I2C Wait Ticks"=w650, "Write Bits Remaining"=w649, "error in (no error)"=w660, "Socket Mask"=w648) -> ("Wait Ticks Remaining Out"=w655:u32, "Procedure Step Out"=w654:T5, "Write Bits Remaining Out"=w653:u8, "Finished"=w658:bool, "error out"=w659:errorcluster)  [unwired: 5 in]
              n136 = Bundle By Name(cluster=w657, "Wait Ticks Remaining"=w655, "Procedure Step"=w654, "Write Bits Remaining"=w653) -> (w656:T11)
            }
            frame "I2C-Read ACK" {
              n137 = call "WSVCAP SHL FPGA LL Procedure I2C - Read ACK.vi"("Procedure Step"=w665, "Wait Ticks Remaining"=w662, "I2C Wait Ticks"=w664, "Socket Mask"=w663, "error in (no error)"=w671) -> ("Wait Ticks Remaining Out"=w661:u32, "Procedure Step Out"=w666:T5, "Finished"=w669:bool, "error out"=w670:errorcluster)  [unwired: 6 in, 1 out]
              n138 = Bundle By Name(cluster=w667, "Wait Ticks Remaining"=w661, "Procedure Step"=w666) -> (w668:T11)
            }
            frame "I2C-Receive Byte" {
              n139 = call "WSVCAP SHL FPGA LL Procedure I2C - Receive Byte.vi"("Procedure Step"=w676, "Wait Ticks Remaining"=w682, "I2C Wait Ticks"=w675, "Read Bits Remaining"=w674, "Read Bytes Remaining"=w673, "error in (no error)"=w686, "Socket Mask"=w672) -> ("Wait Ticks Remaining Out"=w681:u32, "Procedure Step Out"=w679:T5, "Finished"=w680:bool, "Read Bits Remaining Out"=w678:u8, "Read Bytes Remaining Out"=w677:u8, "error out"=w685:errorcluster)  [unwired: 3 in]
              n140 = Bundle By Name(cluster=w684, "Wait Ticks Remaining"=w681, "Procedure Step"=w679, "Read Bits Remaining"=w678, "Read Bytes Remaining"=w677) -> (w683:T11)
            }
            frame "I2C-Write ACK" {
              n141 = Less Or Equal To 0?(x=w687) -> (x <= 0?=w696:bool)
              n142 = call "WSVCAP SHL FPGA LL Procedure I2C - Send ACK.vi"("Procedure Step"=w693, "Wait Ticks Remaining"=w694, "I2C Wait Ticks"=w692, "ACK Bit to Write"=w696, "error in (no error)"=w699, "Socket Mask"=w695) -> ("Wait Ticks Remaining Out"=w689:u32, "Procedure Step Out"=w688:T5, "Finished"=w697:bool, "error out"=w698:errorcluster)  [unwired: 6 in]
              n143 = Bundle By Name(cluster=w691, "Wait Ticks Remaining"=w689, "Procedure Step"=w688) -> (w690:T11)
            }
            frame "SPI-Clear Lines" {
              n144 = Equal?(x=w700, y=WSVCAP_SHL_Operation_Step_Enum."SPI Write/Read - A: SPI-Clear Lines") -> (x = y?=w703:bool)
              n145 = call "WSVCAP SHL FPGA LL Procedure SPI - Clear Lines.vi"("Enable SPI"=w703, "error in (no error)"=w707, "Socket Mask"=w702) -> ("error out"=w706:errorcluster)  [unwired: 12 in]
            }
            frame "SPI-Send/Receive" {
              n146 = call "WSVCAP SHL FPGA LL Procedure SPI - Send Receive.vi"("Procedure Step"=w715, "Wait Ticks Remaining"=w714, "CMD Length [1-40]"=w713, "SPI Wait Ticks"=w708, "Write Bit Index [0-39]"=w716, "SPI Cycle Mode"=w717, "error in (no error)"=w723, "SPI Cycle CMD"=w718, "Socket Mask"=w719) -> ("Wait Ticks Remaining Out"=w712:u32, "Procedure Step Out"=w711:T5, "Write Bit Index [0-39] Out"=w709:u8, "Finished"=w710:bool, "error out"=w722:errorcluster)  [unwired: 2 in]
              n147 = Bundle By Name(cluster=w721, "Wait Ticks Remaining"=w712, "Procedure Step"=w711, "Write Bit Index [0-39]"=w709) -> (w720:T11)
            }
            frame "SPI-Wait CMD Delay" {
              # "First Tick"
              # "Last Tick"
              n148 = Select(t=w736, s=w739, f=w738) -> (s? t:f=w737:u32)
              n149 = Equal?(x=w725, y=w728) -> (x = y?=w727:bool)
              n150 = Decrement(x=w737) -> (x-1=w740:u32)
              n151 = Compound Arithmetic op=AND(w727, w726) -> (w724:bool)
              n152 = Equal?(x=w737, y=w736) -> (x = y?=w732:bool)
              n153 = Less Or Equal To 0?(x=w740) -> (x <= 0?=w730:bool)
              n154 = Bundle By Name(cluster=w734, "Wait Ticks Remaining"=w740) -> (w733:T11)
              n155 = Compound Arithmetic op=AND(w730, invert w724) -> (w729:bool)
              n156 = Compound Arithmetic op=OR(w729, w732) -> (w731:bool)
              n157 = case shown="True" w731 {
                tunnel: w742 -> [w743 w747]
                tunnel: [w743 w746] -> w741
                tunnel: w735 -> [_ w745]
                tunnel: w729 -> [_ w744]
                frame False {
                }
                frame True {
                  # "First or Last Tick of Wait Cycle"
                  n158 = call "WSVCAP SHL FPGA LL Procedure SPI - Clear Lines.vi"("Enable SPI"=w744, "error in (no error)"=w747, "Socket Mask"=w745) -> ("error out"=w746:errorcluster)  [unwired: 12 in]
                }
              }
            }
            frame "RFFE-Wait CMD Delay" {
              # "First Tick"
              n159 = Select(t=w760, s=w748, f=w762) -> (s? t:f=w761:u32)
              n160 = Equal?(x=w750, y=w753) -> (x = y?=w752:bool)
              n161 = Decrement(x=w761) -> (x-1=w763:u32)
              n162 = Compound Arithmetic op=AND(w752, w751) -> (w749:bool)
              n163 = Less Or Equal To 0?(x=w763) -> (x <= 0?=w755:bool)
              n164 = Bundle By Name(cluster=w758, "Wait Ticks Remaining"=w763) -> (w757:T11)
              n165 = Compound Arithmetic op=AND(w755, invert w749) -> (w754:bool)
              n166 = Compound Arithmetic op=OR(w754, w748) -> (w756:bool)
              n167 = case shown="True" w756 {
                tunnel: w765 -> [w766 w769]
                tunnel: [w766 w768] -> w764
                tunnel: w759 -> [_ w767]
                frame False {
                }
                frame True {
                  # "First or Last Tick of Wait Cycle"
                  n168 = call "WSVCAP SHL FPGA LL Procedure RFFE - Clear Lines.vi"("error in (no error)"=w769, "Socket Mask"=w767) -> ("error out"=w768:errorcluster)  [unwired: 13 in]
                }
              }
            }
            frame "RFFE-Clear Lines" {
              n169 = call "WSVCAP SHL FPGA LL Procedure RFFE - Clear Lines.vi"("error in (no error)"=w772, "Socket Mask"=w770) -> ("error out"=w771:errorcluster)  [unwired: 13 in]
            }
            frame "RFFE-Send SSC" {
              n170 = call "WSVCAP SHL FPGA LL Procedure RFFE - Send SSC.vi"("Procedure Step"=w780, "Wait Ticks Remaining"=w779, "Wait Ticks"=w775, "error in (no error)"=w785, "Socket Mask"=w781) -> ("Wait Ticks Remaining Out"=w778:u32, "Procedure Step Out"=w777:T5, "Finished"=w776:bool, "error out"=w784:errorcluster)  [unwired: 7 in]
              n171 = Bundle By Name(cluster=w783, "Wait Ticks Remaining"=w778, "Procedure Step"=w777) -> (w782:T11)
            }
            frame "RFFE-Send Data" {
              n172 = call "WSVCAP SHL FPGA LL Procedure RFFE - Send Data.vi"("Procedure Step"=w794, "Wait Ticks Remaining"=w793, "CMD Length [1-48]"=w792, "RFFE Wait Ticks"=w788, "Write Bit Index [0-47]"=w787, "RFFE Cycle Mode"=w795, "error in (no error)"=w801, "RFFE Cycle CMD"=w796, "Socket Mask"=w797) -> ("Wait Ticks Remaining Out"=w791:u32, "Procedure Step Out"=w790:T5, "Write Bit Index [0-47] Out"=w789:u8, "Finished"=w786:bool, "error out"=w800:errorcluster)  [unwired: 2 in]
              n173 = Bundle By Name(cluster=w799, "Wait Ticks Remaining"=w791, "Procedure Step"=w790, "Write Bit Index [0-39]"=w789) -> (w798:T11)
            }
            frame "RFFE-Receive Data" {
              n174 = call "WSVCAP SHL FPGA LL Procedure RFFE - Receive Data.vi"("Procedure Step"=w812, "Wait Ticks Remaining"=w811, "Start of Procedure"=w804, "RFFE Wait Ticks"=w806, "Read Bits Remaining"=w805, "Read Bytes Remaining"=w803, "error in (no error)"=w818, "RFFE Cycle CMD"=w813, "Socket Mask"=w814) -> ("Wait Ticks Remaining Out"=w810:u32, "Procedure Step Out"=w809:T5, "Read Bytes Remaining Out"=w802:u8, "Read Bits Remaining Out"=w807:u8, "Finished"=w808:bool, "error out"=w817:errorcluster)  [unwired: 1 in]
              n175 = Bundle By Name(cluster=w816, "Wait Ticks Remaining"=w810, "Procedure Step"=w809, "Read Bytes Remaining"=w802, "Read Bits Remaining"=w807) -> (w815:T11)
            }
          }
          n176 = case "Post-Procedure" shown="\"RFFE Write Data - B: Send Data\"" w383 {
            selector: w383 -> [w460 w463 w468 w469 w473 w477 w480 _ w487 w500 w501 w505 w507 w517 w521 w526 w528 w558 w560 w566 w571 w574 w579 w597 w612 w615]
            tunnel: [w458 w462 w466 w470 w474 w479 w482 w484 w489 w496 w503 w506 w511 w520 w523 w527 w546 w559 w562 w568 w573 w576 w581 w601 w613 w616] -> w407
            tunnel: w409 -> [w458 w462 w466 w470 w474 w479 w482 w484 w489 w497 w503 w506 w511 w520 w523 w527 w546 w559 w562 w568 w573 w576 w581 w601 w613 w616]
            tunnel: [_ _ _ w471 _ _ w481 _ _ _ w502 _ _ _ w522 _ _ _ w561 _ _ w575 _ _ _ w614] -> w401
            tunnel: w402 -> [w457 _ w465 w471 _ w476 w481 _ w485 w498 w502 _ w509 w519 w522 _ w538 w549 w561 w565 w569 w575 w577 w591 w605 w614]
            tunnel: [w456 w461 w464 w469 w472 w475 w480 WSVCAP_SHL_Operation_Step_Enum."I2C Send Data - B: Send Data Byte" ("Operation Step") w486 w499 w501 w504 w508 w518 w521 w525 w545 w557 w560 w564 w570 w574 w578 w600 w611 w615] -> w403
            tunnel: [_ _ _ _ _ _ _ _ _ _ _ _ _ _ _ TRUE ("Finished") w539 w547 _ TRUE ("Finished") _ _ w577 w592 _ _] -> w408
            tunnel: w389 -> [_ _ _ _ _ _ _ _ _ _ _ _ _ _ _ _ w535 _ _ _ _ _ _ w588 _ _]
            tunnel: w388 -> [_ _ _ _ _ _ _ _ _ _ _ _ _ _ _ _ w537 _ _ _ _ _ _ w590 _ _]
            tunnel: "Stop Cycle" -> [_ _ _ _ _ _ _ _ _ _ _ _ _ _ _ _ w531 w550 _ _ _ _ _ w582 w604 _]
            tunnel: w384 -> [_ _ _ _ _ _ _ _ _ _ _ _ _ _ _ _ w534 w552 _ _ _ _ _ w587 w607 _]
            tunnel: w385 -> [_ _ _ _ _ _ _ _ _ _ _ _ _ _ _ _ w533 w551 _ _ _ _ _ w586 w606 _]
            tunnel: w381 -> [_ _ _ _ _ _ _ _ _ _ _ _ _ w512 _ _ _ _ _ _ _ _ _ _ _ _]
            frame "I2C Send Slave Add - A: Send Start Sequence" {
              n177 = Increment(x=w460) -> (x+1=w459:T6)
              n178 = Select(t=w459, s=w457, f=w460) -> (s? t:f=w456:T6)
            }
            frame "I2C Send Slave Add - B: Load Address Byte" {
              n179 = Increment(x=w463) -> (x+1=w461:T6)
            }
            frame "I2C Send Slave Add - C: Send Address Byte" {
              n180 = Increment(x=w468) -> (x+1=w467:T6)
              n181 = Select(t=w467, s=w465, f=w468) -> (s? t:f=w464:T6)
            }
            frame "I2C Send Slave Add - D: Read Slave ACK" {
            }
            frame "I2C Send Sub Add - A: Load Sub Address" {
              n182 = Increment(x=w473) -> (x+1=w472:T6)
            }
            frame "I2C Send Sub Add - B: Send Address Byte" {
              n183 = Increment(x=w477) -> (x+1=w478:T6)
              n184 = Select(t=w478, s=w476, f=w477) -> (s? t:f=w475:T6)
            }
            frame "I2C Send Sub Add - C: Read Slave ACK" {
            }
            frame "I2C Send Data - A: Get Byte from FIFO" {
            }
            frame "I2C Send Data - B: Send Data Byte" {
              n185 = Increment(x=w487) -> (x+1=w488:T6)
              n186 = Select(t=w488, s=w485, f=w487) -> (s? t:f=w486:T6)
            }
            frame "I2C Send Data - C: Read Slave ACK" {
              n187 = call "WSVCAP SHL FPGA LL I2C FIFO Manager - Transfer.vi"("error in (no error)"=w497, "Operation"=WSVCAP_SHL_FIFO_Operation_Enum."Get Write FIFO Status") -> ("Data Out"=w494:u64, "error out"=w496:errorcluster)  [unwired: 11 in, 1 out]
              n188 = Equal To 0?(x=w494) -> (x = 0?=w493:bool)
              n189 = Select(t=WSVCAP_SHL_Operation_Step_Enum."I2C Send Data - D: Send Stop Sequence" ("Operation Step"), s=w493, f=WSVCAP_SHL_Operation_Step_Enum."I2C Send Data - A: Get Byte from FIFO" ("Operation Step")) -> (s? t:f=w490:T6)
              n190 = Select(t=w490, s=w498, f=w500) -> (s? t:f=w499:T6)
            }
            frame "I2C Send Data - D: Send Stop Sequence" {
            }
            frame "I2C Read Data - A: Load Bytes to Read" {
              n191 = Increment(x=w505) -> (x+1=w504:T6)
            }
            frame "I2C Read Data - B: Receive Byte" {
              n192 = Increment(x=w507) -> (x+1=w510:T6)
              n193 = Select(t=w510, s=w509, f=w507) -> (s? t:f=w508:T6)
            }
            frame "I2C Read Data - C: Write Master ACK" {
              n194 = Less Or Equal To 0?(x=w512) -> (x <= 0?=w513:bool)
              n195 = Increment(x=w517) -> (x+1=w515:T6)
              n196 = Select(t=w515, s=w513, f=WSVCAP_SHL_Operation_Step_Enum."I2C Read Data - B: Receive Byte" ("Operation Step")) -> (s? t:f=w514:T6)
              n197 = Select(t=w514, s=w519, f=w517) -> (s? t:f=w518:T6)
            }
            frame "I2C Read Data - D: Send Stop Sequence" {
            }
            frame "SPI Write/Read - A: SPI-Clear Lines" {
              # "Load First CMD"
              n198 = Increment(x=w526) -> (x+1=w525:T6)
            }
            frame "SPI Write/Read - B: SPI-Send/Receive Data" {
              n199 = Equal To 0?(x=w535) -> (x = 0?=w529:bool)
              n200 = Equal?(x=w534, y=w533) -> (x = y?=w532:bool)
              n201 = Compound Arithmetic op=AND(w532, w531) -> (w530:bool)
              n202 = Select(t=w528, s=w529, f=WSVCAP_SHL_Operation_Step_Enum."SPI Write/Read - C: SPI-Wait CMD Delay" ("Operation Step")) -> (s? t:f=w541:T6)
              n203 = Select(t=WSVCAP_SHL_Operation_Step_Enum."SPI Write/Read - D:SPI-Clear Lines" ("Operation Step"), s=w530, f=w541) -> (s? t:f=w540:T6)
              n204 = Select(t=w540, s=w537, f=WSVCAP_SHL_Operation_Step_Enum."SPI Write/Read - D:SPI-Clear Lines" ("Operation Step")) -> (s? t:f=w544:T6)
              n205 = Compound Arithmetic op=AND(invert w530, w529, w537, w538) -> (w539:bool)
              n206 = Select(t=w544, s=w538, f=w528) -> (s? t:f=w545:T6)
            }
            frame "SPI Write/Read - C: SPI-Wait CMD Delay" {
              n207 = Equal?(x=w552, y=w551) -> (x = y?=w553:bool)
              n208 = Compound Arithmetic op=AND(w550, w553) -> (w548:bool)
              n209 = Select(t=WSVCAP_SHL_Operation_Step_Enum."SPI Write/Read - D:SPI-Clear Lines" ("f"), s=w548, f=WSVCAP_SHL_Operation_Step_Enum."SPI Write/Read - B: SPI-Send/Receive Data") -> (s? t:f=w555:T6)
              n210 = Compound Arithmetic op=AND(invert w548, w549) -> (w547:bool)
              n211 = Select(t=w555, s=w549, f=w558) -> (s? t:f=w557:T6)
            }
            frame "SPI Write/Read - D:SPI-Clear Lines" {
            }
            frame "RFFE Read Data - A: Send SSC" {
              n212 = Increment(x=w566) -> (x+1=w567:T6)
              n213 = Select(t=w567, s=w565, f=w566) -> (s? t:f=w564:T6)
            }
            frame "RFFE Read Data - B: Send CMD Frame" {
              n214 = Increment(x=w571) -> (x+1=w572:T6)
              n215 = Select(t=w572, s=w569, f=w571) -> (s? t:f=w570:T6)
            }
            frame "RFFE Read Data - C: Receive Byte" {
            }
            frame "RFFE Write Data - A: Send SSC" {
              n216 = Increment(x=w579) -> (x+1=w580:T6)
              n217 = Select(t=w580, s=w577, f=w579) -> (s? t:f=w578:T6)
            }
            frame "RFFE Write Data - B: Send Data" {
              n218 = Equal To 0?(x=w588) -> (x = 0?=w583:bool)
              n219 = Equal?(x=w587, y=w586) -> (x = y?=w585:bool)
              n220 = Compound Arithmetic op=AND(w585, w582) -> (w584:bool)
              n221 = Select(t=WSVCAP_SHL_Operation_Step_Enum."RFFE Write Data - A: Send SSC" ("Operation Step"), s=w583, f=WSVCAP_SHL_Operation_Step_Enum."RFFE Write Data - C: Wait CMD Delay" ("Operation Step")) -> (s? t:f=w594:T6)
              n222 = Select(t=WSVCAP_SHL_Operation_Step_Enum."RFFE Write Data - D: Clear Lines" ("Operation Step"), s=w584, f=w594) -> (s? t:f=w593:T6)
              n223 = Select(t=w593, s=w590, f=WSVCAP_SHL_Operation_Step_Enum."RFFE Write Data - D: Clear Lines" ("Operation Step")) -> (s? t:f=w599:T6)
              n224 = Compound Arithmetic op=AND(w584, w590, w591) -> (w592:bool)
              n225 = Select(t=w599, s=w591, f=w597) -> (s? t:f=w600:T6)
            }
            frame "RFFE Write Data - C: Wait CMD Delay" {
              n226 = Equal?(x=w607, y=w606) -> (x = y?=w603:bool)
              n227 = Compound Arithmetic op=AND(w604, w603) -> (w602:bool)
              n228 = Select(t=WSVCAP_SHL_Operation_Step_Enum."RFFE Write Data - D: Clear Lines" ("f"), s=w602, f=WSVCAP_SHL_Operation_Step_Enum."RFFE Write Data - A: Send SSC") -> (s? t:f=w609:T6)
              n229 = Select(t=w609, s=w605, f=w612) -> (s? t:f=w611:T6)
            }
            frame "RFFE Write Data - D: Clear Lines" {
            }
          }
          n230 = case shown="True" w408 {
            tunnel: w387 -> [w452 w455]
            tunnel: [w452 w454] -> w406
            frame False {
            }
            frame True {
              # "Load next SPI or RFFE\nCycle CMD"
              n231 = call "WSVCAP SHL FPGA LL RFFE Load Next Cycle CMD.vi"("Transfer Cluster In"=w455) -> ("Transfer Cluster Out"=w454:T11, "SPI Cycle Count"=→"Cycle Count":u64)  [unwired: 13 in]
            }
          }
          n232 = case "Post Operation" shown="\"RFFE Ext Read - I:Read Data\"" w414 {
            selector: w414 -> [w422 w426 w429 w432 w436 w440 w445 w446 w449 w451]
            tunnel: [_ _ w428 _ _ _ w444 w447 w448 w450] -> w416
            tunnel: w401 -> [w420 w424 w428 w431 w435 w439 w444 w447 w448 w450]
            tunnel: [w423 w427 w429 w430 w434 w438 w442 w446 w449 w451] -> w404
            frame "I2C Write - I:Send Slave Address" {
              n233 = Increment(x=w422) -> (x+1=w421:T7)
              n234 = Select(t=w421, s=w420, f=w422) -> (s? t:f=w423:T7)
            }
            frame "I2C Write - II:Send Sub Address" {
              n235 = Increment(x=w426) -> (x+1=w425:T7)
              n236 = Select(t=w425, s=w424, f=w426) -> (s? t:f=w427:T7)
            }
            frame "I2C Write - III:Send Data Bytes" {
            }
            frame "I2C Read - I:Send Slave Address (W)" {
              n237 = Increment(x=w432) -> (x+1=w433:T7)
              n238 = Select(t=w433, s=w431, f=w432) -> (s? t:f=w430:T7)
            }
            frame "I2C Read - II:Send Sub Address" {
              n239 = Increment(x=w436) -> (x+1=w437:T7)
              n240 = Select(t=w437, s=w435, f=w436) -> (s? t:f=w434:T7)
            }
            frame "I2C Read - III:Send Slave Address (R)" {
              n241 = Increment(x=w440) -> (x+1=w441:T7)
              n242 = Select(t=w441, s=w439, f=w440) -> (s? t:f=w438:T7)
            }
            frame "I2C Read - IV:Read Data Bytes" {
              n243 = Select(t=WSVCAP_SHL_Transaction_Step_Enum."I2C Read - I:Send Slave Address (W)" ("Transaction Step"), s=w444, f=w445) -> (s? t:f=w442:T7)
            }
            frame "SPI Write/Read - I:SPI-Write/Read Data" {
            }
            frame "RFFE Ext Write - I.Write Data" {
            }
            frame "RFFE Ext Read - I:Read Data" {
            }
          }
          n244 = Bundle By Name(cluster=w406, "Transaction Step"=w404, "Operation Step"=w403, "Start Operation"=w401, "Start Procedure"=w402) -> (w405:T11)
          n245 = disable-structure shown="TARGET_TYPE!=FPGA, default" {
            disable-tunnel: w415 -> [w819 _]
            disable-tunnel: w416 -> [_ _]
            frame condition #0 (active) {
              n246 = case shown="\"RFFE-Ext Write\", \"RFFE-Ext Read\"" w819 {
                tunnel: [w824 w837 w846] -> w820
                frame "SPI-Write/Read Data" {
                  n247 = global read "WSVCAP SHL FPGA LL SPI Debug Global.vi" "SPI_CLK"() -> (w823:bool)
                  n248 = global read "WSVCAP SHL FPGA LL SPI Debug Global.vi" "SPI_DAA"() -> (w822:bool)
                  n249 = global read "WSVCAP SHL FPGA LL SPI Debug Global.vi" "SPI_EN"() -> (w821:bool)
                  n250 = global read "WSVCAP SHL FPGA LL SPI Debug Global.vi" "SPI_DATO"() -> (w828:bool)
                  n251 = Boolean To (0,1)(Boolean=w823) -> (0, 1=w831:i16)
                  n252 = Boolean To (0,1)(Boolean=w822) -> (0, 1=w830:i16)
                  n253 = Boolean To (0,1)(Boolean=w821) -> (0, 1=w829:i16)
                  n254 = Boolean To (0,1)(Boolean=w828) -> (0, 1=w827:i16)
                  n255 = Bundle(w831, w830, w829, w827) -> (w826:cluster{i16, i16, i16, i16})  [unwired: 1 in]
                  n256 = Add(x=w826, y=cluster{i16, i16, i16, i16} {0, 2, 4, 6} ("Waveform Chart")) -> (x+y=w824:cluster{i16, i16, i16, i16})
                }
                frame "RFFE-Ext Write", "RFFE-Ext Read" {
                  n257 = global read "WSVCAP SHL FPGA LL RFFE Debug Global.vi" "RFFE_CLK"() -> (w836:bool)
                  n258 = global read "WSVCAP SHL FPGA LL RFFE Debug Global.vi" "RFFE_DAA"() -> (w835:bool)
                  n259 = global read "WSVCAP SHL FPGA LL RFFE Debug Global.vi" "RFFE_CLK"() -> (w840:bool)
                  n260 = global read "WSVCAP SHL FPGA LL RFFE Debug Global.vi" "RFFE_DATO"() -> (w833:bool)
                  n261 = Boolean To (0,1)(Boolean=w836) -> (0, 1=w842:i16)
                  n262 = Boolean To (0,1)(Boolean=w835) -> (0, 1=w841:i16)
                  n263 = Boolean To (0,1)(Boolean=w840) -> (0, 1=w834:i16)
                  n264 = Boolean To (0,1)(Boolean=w833) -> (0, 1=w832:i16)
                  n265 = Bundle(w842, w841, w834, w832) -> (w839:cluster{i16, i16, i16, i16})  [unwired: 1 in]
                  n266 = Add(x=w839, y=cluster{i16, i16, i16, i16} {0, 2, 4, 6} ("Waveform Chart")) -> (x+y=w837:cluster{i16, i16, i16, i16})
                }
                frame Default {
                  w845 = i16 0 ("0, 1")
                  n267 = global read "WSVCAP SHL FPGA LL I2C Debug Global.vi" "I2C SCL"() -> (w844:bool)
                  n268 = global read "WSVCAP SHL FPGA LL I2C Debug Global.vi" "I2C SDA"() -> (w843:bool)
                  n269 = Boolean To (0,1)(Boolean=w844) -> (0, 1=w850:i16)
                  n270 = Boolean To (0,1)(Boolean=w843) -> (0, 1=w849:i16)
                  n271 = Bundle(w850, w849, "0, 1"=w845, "0, 1"=w845) -> (w848:cluster{i16, i16, "0, 1":i16, "0, 1":i16})  [unwired: 1 in]
                  n272 = Add(x=w848, y=cluster{i16, i16, i16, i16} {0, 2, -1, -1} ("Waveform Chart")) -> (x+y=w846:cluster{i16, i16, i16, i16})
                }
              }
              "Waveform Chart" <- w820
            }
            frame condition #1 {
            }
          }
          n273 = Unbundle By Name(w407) -> ("status"=w419:bool)
          n274 = To Long Integer(number=w415) -> (32bit integer=w417:i32)
          n275 = Compound Arithmetic op=OR(w416, w419) -> (w418:bool)
        }
        n276 = node-c288(w378) -> ()
      }
      frame "Post Transmition" {
        # "1 Second (Ticks)"
        # "Error Info"
        # "Transfer Data from Read FIFO to Host"
        n277 = Unbundle By Name(w859) -> ("Cycle Count"=w856:u64, "Cycle Mode"=w857:bool, "Bytes to Read"=w861:u8, "Transaction"=w865:T1)
        n278 = Increment(x=w856) -> (x+1=w860:u64)
        n279 = Select(t=w860, s=w857, f=w856) -> (s? t:f=w855:u64)
        n280 = Bundle By Name(cluster=w859, "Cycle Count"=w855) -> (w858:T11)
        n281 = case shown="..0" w861 {
          selector: w861 -> [_ w871]
          tunnel: w867 -> [w870 w879]
          tunnel: [w870 w878] -> w866
          tunnel: w865 -> [_ w875]
          tunnel: w864 -> [_ w874]
          tunnel: [w869 w873] -> w863
          tunnel: w862 -> [w869 w872]
          frame ..0 {
            # "No Read Operation"
          }
          frame 1.. {
            # "Transfer Read Data"
            # "Read all data and transfer to the host"
            n282 = Multiply(x=w871, y=u8 8) -> (x*y=w877:u8)
            n283 = To Long Integer(number=w877) -> (32bit integer=w880:i32)
            n284 = for {
              N: w880 -> [_]
              shift-right: [w896] -> w878
              shift-left: w879 -> [w897]
              tunnel: w875 -> [w893]
              tunnel: w874 -> [w892]
              shift-right: [w883] -> w873
              shift-left: w872 -> [w881]
              i -> [w886]
              n285 = flat-sequence {
                tunnel: w897 -> [w904]
                tunnel: [w903] -> w894
                tunnel: w893 -> [w901]
                tunnel: w892 -> [w900]
                tunnel: [w900] -> w891
                tunnel: [w899] -> w887
                tunnel: w886 -> [w899]
                tunnel: [w898] -> w884
                tunnel: w881 -> [w898]
                tunnel: [w922] -> w895
                tunnel: w894 -> [w922]
                tunnel: w891 -> [w921]
                tunnel: [w921] -> w890
                tunnel: [w920] -> w888
                tunnel: w887 -> [w920]
                tunnel: [w919] -> w885
                tunnel: w884 -> [w919]
                tunnel: w895 -> [w931]
                tunnel: w890 -> [w932]
                tunnel: [w930] -> w889
                tunnel: w888 -> [w926]
                tunnel: w885 -> [w925]
                tunnel: [w924] -> w882
                tunnel: [w952] -> w896
                tunnel: w889 -> [w952]
                tunnel: [w951] -> w883
                tunnel: w882 -> [w951]
                frame #0 {
                  n286 = case shown="\"RFFE-Ext Write\", \"RFFE-Ext Read\"" w901 {
                    tunnel: w904 -> [w908 w913 w918]
                    tunnel: [w907 w912 w917] -> w903
                    tunnel: [w906 w909 w914] -> w902
                    frame "I2C-Read Data", "I2C-Write Data" {
                      n287 = call "WSVCAP SHL FPGA LL I2C FIFO Manager - Pre and Post.vi"("error in (no error)"=w908, "Operation"=WSVCAP_SHL_FIFO_Operation_Enum."Get Element from Read") -> ("64 Bit Data Out"=w906:u64, "error out"=w907:errorcluster)  [unwired: 11 in, 1 out]
                    }
                    frame "SPI-Write/Read Data" {
                      n288 = call "WSVCAP SHL FPGA LL SPI FIFO Manager - Pre and Post.vi"("error in (no error)"=w913, "Operation"=WSVCAP_SHL_FIFO_Operation_Enum."Get Element from Read") -> ("Word Out"=w911:u16, "error out"=w912:errorcluster)  [unwired: 11 in, 1 out]
                      n289 = To Unsigned Quad Integer(1:w911) -> (0:w909:u64)
                    }
                    frame "RFFE-Ext Write", "RFFE-Ext Read" {
                      n290 = call "WSVCAP SHL FPGA LL RFFE FIFO Manager - Pre and Post.vi"("error in (no error)"=w918, "Operation"=WSVCAP_SHL_FIFO_Operation_Enum."Get Element from Read") -> ("Word Out"=w916:u16, "error out"=w917:errorcluster)  [unwired: 11 in, 1 out]
                      n291 = To Unsigned Quad Integer(1:w916) -> (0:w914:u64)
                    }
                  }
                  "Read Data" <- w902
                }
                frame #1 {
                  "Read Flag" <- TRUE ("Read Flag")
                }
                frame #2 {
                  n292 = call "Tick Count2"() -> ("Tick Count(mSec)"=w933:u32)
                  n293 = while {
                    tunnel: w933 -> [w948]
                    tunnel: w932 -> [w946]
                    tunnel: w931 -> [w945]
                    tunnel: ["Ack Read"] -> w928
                    tunnel: [w942] -> w929
                    stop <- w943 stop-if-true
                    n294 = Unbundle By Name(w945) -> ("status"=w944:bool)
                    n295 = call "Wait2"("Count(mSec)"=u32 1 ("Count(Ticks)")) -> ("Tick Count(mSec)"=w949:u32)
                    n296 = Subtract(x=w949, y=w948) -> (x-y=w947:u32)
                    n297 = Greater?(x=w947, y=w946) -> (0:w942:bool)
                    n298 = Compound Arithmetic op=OR(w944, w942, "Ack Read") -> (w943:bool)
                  }
                  n299 = Compound Arithmetic op=AND(w929, invert w928) -> (w927:bool)
                  n300 = case shown="False" w927 {
                    selector: w927 -> [_ w939]
                    tunnel: [w935 w938] -> w930
                    tunnel: w931 -> [w935 w940]
                    tunnel: [w934 w936] -> w924
                    tunnel: w926 -> [_ w936]
                    tunnel: w925 -> [w934 _]
                    frame False {
                    }
                    frame True {
                      n301 = Bundle By Name(cluster=w940, "status"=w939, "code"=9902) -> (w938:errorcluster)
                    }
                  }
                }
                frame #3 {
                  n302 = local write "Ack Read"(FALSE ("Read Flag")) -> ()
                }
              }
            }
          }
        }
      }
      frame "Operation Complete" {
        # "Transfer Status"
        n303 = Unbundle By Name(w955) -> ("Cycle Mode"=w954:bool)
        n304 = To Long Integer(number=w959) -> (32bit integer=w958:i32)
        n305 = case shown="False" w954 {
          tunnel: w960 -> [w967 _]
          tunnel: w958 -> [w966 _]
          tunnel: w957 -> [w965 _]
          tunnel: w956 -> [w963 _]
          frame False {
            # "Return Status"
            n306 = for {
              N: 4 -> [_]
              tunnel: w967 -> [w974]
              tunnel: w966 -> [w973]
              tunnel: w965 -> [w972]
              tunnel: w963 -> [w968]
              i -> [w971]
              n307 = flat-sequence {
                tunnel: w974 -> [w984]
                tunnel: w973 -> [w977]
                tunnel: w972 -> [w976]
                tunnel: w971 -> [w981]
                tunnel: [w975] -> w969
                tunnel: w968 -> [w975]
                tunnel: [w989] -> w970
                tunnel: w969 -> [w989]
                tunnel: w970 -> [w991]
                frame #0 {
                  # "Iteration"
                  # "Error Info"
                  # "Last State"
                  # "Error Code"
                  # "Error Status"
                  n308 = Unbundle By Name(w984) -> ("status"=w983:bool, "code"=w978:i32)
                  n309 = Boolean To (0,1)(Boolean=w983) -> (0, 1=w982:i16)
                  n310 = To Long Integer(number=w982) -> (32bit integer=w980:i32)
                  n311 = case shown="3" w981 {
                    tunnel: [w985 w986 w987 w988] -> w979
                    tunnel: w980 -> [w985 _ _ _]
                    tunnel: w978 -> [_ w986 _ _]
                    tunnel: w977 -> [_ _ w987 _]
                    tunnel: w976 -> [_ _ _ w988]
                    frame Default {
                    }
                    frame 1 {
                    }
                    frame 2 {
                    }
                    frame 3 {
                    }
                  }
                  "Status" <- w979
                }
                frame #1 {
                  "Read Status Flag" <- TRUE ("Read Flag")
                }
                frame #2 {
                  n312 = call "Tick Count3"() -> ("Tick Count(mSec)"=w992:u32)
                  n313 = while {
                    tunnel: w992 -> [w998]
                    tunnel: w991 -> [w996]
                    stop <- w995 stop-if-true
                    n314 = call "Wait3"("Count(mSec)"=u32 1 ("Count(Ticks)")) -> ("Tick Count(mSec)"=w999:u32)
                    n315 = Subtract(x=w999, y=w998) -> (x-y=w997:u32)
                    n316 = Greater?(x=w997, y=w996) -> (0:w994:bool)
                    n317 = Compound Arithmetic op=OR(w994, "Ack Read Status") -> (w995:bool)
                  }
                }
                frame #3 {
                  n318 = local write "Ack Read Status"(FALSE ("Read Flag")) -> ()
                }
              }
            }
          }
          frame True {
            # "No Status from Cycle Mode"
          }
        }
        n319 = local write "Cmd"(WSVCAP_SHL_State."Idle" ("SPI_CMD_DBG")) -> ()
      }
    }
    n320 = Select(t=WSVCAP_SHL_Communication_Loop_State."Operation Complete" ("Action"), s=w19, f=w21) -> (s? t:f=w20:T3)
  }
  n321 = local write "Exit"(w4) -> ()
